vi "Lockin-4461 -Patrick -State -sw_timed_single_pt.vi"() -> ()   [LabVIEW 2013]
uses:
  <vilib>/Analysis/4window.llb/windowTd.ctl
  <vilib>/measure/maspectr.llb/Power Spectrum and PSD Export Mode.ctl
  <vilib>/Utility/error.llb/DialogType.ctl
  <vilib>/Analysis/baseanly.llb/Mean (DBL).vi
  <vilib>/Analysis/2dsp.llb/Decimate (single shot).vi
  <vilib>/Analysis/2dsp.llb/Decimate (single shot, DBL).vi
  <userlib>/_OpenG.lib/array/array.llb/Empty 1D Array (Variant)__ogtk.vi
  <userlib>/_OpenG.lib/array/array.llb/Empty 1D Array (DBL)__ogtk.vi
  <vilib>/measure/maspectr.llb/FFT Power Spectrum and PSD for N Chan.vi
  <vilib>/Waveform/WDTOps.llb/WDT Waveform to XY Pairs DBL.vi
  <vilib>/measure/NI_MAPro.lvlib
  <vilib>/Analysis/NI_AALBase.lvlib
  <vilib>/platform/TimedLoop/XDataNode/XDataNode.xnode
  <vilib>/Platform/TimedLoop/XDataNode/nitl_modes.ctl
  <vilib>/Platform/TimedLoop/XDataNode/XDNodeRunTimeDep.lvlib
  <vilib>/Platform/TimedLoop/XDataNode/wakeup.ctl
  <vilib>/Platform/TimedLoop/XDataNode/timing_clust.ctl
  <vilib>/Analysis/NI_AALPro.lvlib
panel:
  in  "save interval (s)":dbl=300.0
  out "save time":timestamp
  out "Error":bool
  out "Results\n(X, Y, R, Theta, mean)":dbl[][](array[numeric])=[[0.808038444568405, -0.03366600088138751, 0.8087394682565412, -2.3857835167729093, -0.00016707925782300797], [9.627554098594765e-06, 5.490802829917109e-06, 1.1083262770429771e-05, 29.69704943130355, -2.2076368724747004e-05], [-0.00010109394038729712, -3.9229110623141134e-05, 0.00010843849825275628, -158.79145052912693, -4.4533407950990875e-05], [0.00012303597772851785, 8.954846359566259e-06, 0.00012336142463888693, 4.162780801361146, -2.013001476212871e-05], [-0.00010354663772943155, 3.541276214228395e-05, 0.00010943477467247838, 161.11940514883716, -0.0003907411187114377], [-2.8426533993272308e-05, 9.227244974626337e-05, 9.655191772848101e-05, 107.1225864279026, 0.00020962577788662882], [-5.4970263568529676e-05, 3.5314916918015216e-05, 6.533661480150268e-05, 147.28182071959253, -3.9837928959940376e-05], [0.00011632495217069192, 2.1805466214220965e-05, 0.00011835105768151502, 10.617056167129062, 7.22324246932892e-05], [0.808038444568405, -0.03366600088138751, 0.8087394682565412, -2.3857835167729093, 0.0], [9.627554098594765e-06, 5.490802829917109e-06, 1.1083262770429771e-05, 29.69704943130355, 0.0], [-0.00010109394038729712, -3.9229110623141134e-05, 0.00010843849825275628, -158.79145052912693, 0.0], [0.00012303597772851785, 8.954846359566259e-06, 0.00012336142463888693, 4.162780801361146, 0.0], [-0.00010354663772943155, 3.541276214228395e-05, 0.00010943477467247838, 161.11940514883716, 0.0], [-2.8426533993272308e-05, 9.227244974626337e-05, 9.655191772848101e-05, 107.1225864279026, 0.0], [-5.4970263568529676e-05, 3.5314916918015216e-05, 6.533661480150268e-05, 147.28182071959253, 0.0], [0.00011632495217069192, 2.1805466214220965e-05, 0.00011835105768151502, 10.617056167129062, 0.0]] format="%#_3p"
  out "current time":timestamp=timestamp(3547736420.9269166 s since 1904-01-01)
  in  "Channel":dbl min=0.0 max=7.0 step=1.0
  in  "Display":enum16{"X and Y", "R and Theta"}(ring)
  out "Y or Theta":dbl=-0.03366600088138751 caption="Y or Theta: Current (A) or Voltage (V)" format="%.3p"
  out "X or R":dbl=0.808038444568405 caption="X or R: Current (A) or Voltage (V)" format="%#.3p"
  in  "Save Data":bool
  in  "RESET":bool
  in  "EXIT":bool
  in  "path":path=path "C:/Data/lockin"
  in  "Notes":string
  in  "mean":dbl[](array[numeric])=[-7.421439795208782e-05, -0.00022642109497774898, -0.00010801336111838228, -0.0001940739070778859, -0.00016525478307431987, 0.00040119220463992125, -0.0005006815886623466, 0.00022102245437355468]
  in  "Tab Control 2":T1(tab)
  out "Signals Graph 2":waveform(dbl)[](graph)=[{"t0"=timestamp(3547736422.7899165 s since 1904-01-01), "dt"=4.8828125e-06, "Y"=array[2048 elements]}, {"t0"=timestamp(3547736422.7899165 s since 1904-01-01), "dt"=4.8828125e-06, "Y"=array[2048 elements]}, {"t0"=timestamp(3547736422.7899165 s since 1904-01-01), "dt"=4.8828125e-06, "Y"=array[2048 elements]}, {"t0"=timestamp(3547736422.7899165 s since 1904-01-01), "dt"=4.8828125e-06, "Y"=array[2048 elements]}, {"t0"=timestamp(3547736422.7899165 s since 1904-01-01), "dt"=4.8828125e-06, "Y"=array[2048 elements]}, {"t0"=timestamp(3547736422.7899165 s since 1904-01-01), "dt"=4.8828125e-06, "Y"=array[2048 elements]}, {"t0"=timestamp(3547736422.7899165 s since 1904-01-01), "dt"=4.8828125e-06, "Y"=array[2048 elements]}, {"t0"=timestamp(3547736422.7899165 s since 1904-01-01), "dt"=4.8828125e-06, "Y"=array[2048 elements]}]
  out "Signals Graph":waveform(dbl)[](graph)=[{"t0"=timestamp(3547736419.2449164 s since 1904-01-01), "dt"=4.8828125e-05, "Y"=array[20480 elements]}, {"t0"=timestamp(3547736419.2449164 s since 1904-01-01), "dt"=4.8828125e-05, "Y"=array[20480 elements]}, {"t0"=timestamp(3547736419.2449164 s since 1904-01-01), "dt"=4.8828125e-05, "Y"=array[20480 elements]}, {"t0"=timestamp(3547736419.2449164 s since 1904-01-01), "dt"=4.8828125e-05, "Y"=array[20480 elements]}, {"t0"=timestamp(3547736419.2449164 s since 1904-01-01), "dt"=4.8828125e-05, "Y"=array[20480 elements]}, {"t0"=timestamp(3547736419.2449164 s since 1904-01-01), "dt"=4.8828125e-05, "Y"=array[20480 elements]}, {"t0"=timestamp(3547736419.2449164 s since 1904-01-01), "dt"=4.8828125e-05, "Y"=array[20480 elements]}, {"t0"=timestamp(3547736419.2449164 s since 1904-01-01), "dt"=4.8828125e-05, "Y"=array[20480 elements]}]
  out "Reference Graph":waveform(dbl)[](graph)=[{"t0"=timestamp(3547736419.2449164 s since 1904-01-01), "dt"=4.8828125e-05, "Y"=array[20480 elements]}, {"t0"=timestamp(3547736419.2449164 s since 1904-01-01), "dt"=4.8828125e-05, "Y"=array[20480 elements]}, {"t0"=timestamp(3547736419.2449164 s since 1904-01-01), "dt"=4.8828125e-05, "Y"=array[20480 elements]}, {"t0"=timestamp(3547736419.2449164 s since 1904-01-01), "dt"=4.8828125e-05, "Y"=array[20480 elements]}, {"t0"=timestamp(3547736419.2449164 s since 1904-01-01), "dt"=4.8828125e-05, "Y"=array[20480 elements]}, {"t0"=timestamp(3547736419.2449164 s since 1904-01-01), "dt"=4.8828125e-05, "Y"=array[20480 elements]}, {"t0"=timestamp(3547736419.2449164 s since 1904-01-01), "dt"=4.8828125e-05, "Y"=array[20480 elements]}, {"t0"=timestamp(3547736419.2449164 s since 1904-01-01), "dt"=4.8828125e-05, "Y"=array[20480 elements]}]
  in  "decimate graph":i32=1
  in  "Display n?":bool
  out "Display X (or R)":waveform(dbl)[](graph)=[{"t0"=timestamp(3547736419.2449164 s since 1904-01-01), "dt"=1.0, "Y"=[0.808038444568405]}, {"t0"=timestamp(3547736419.2449164 s since 1904-01-01), "dt"=1.0, "Y"=[9.627554098594765e-06]}, {"t0"=timestamp(3547736419.2449164 s since 1904-01-01), "dt"=1.0, "Y"=[-0.00010109394038729712]}, {"t0"=timestamp(3547736419.2449164 s since 1904-01-01), "dt"=1.0, "Y"=[0.00012303597772851785]}, {"t0"=timestamp(3547736419.2449164 s since 1904-01-01), "dt"=1.0, "Y"=[-0.00010354663772943155]}, {"t0"=timestamp(3547736419.2449164 s since 1904-01-01), "dt"=1.0, "Y"=[-2.8426533993272308e-05]}, {"t0"=timestamp(3547736419.2449164 s since 1904-01-01), "dt"=1.0, "Y"=[-5.4970263568529676e-05]}, {"t0"=timestamp(3547736419.2449164 s since 1904-01-01), "dt"=1.0, "Y"=[0.00011632495217069192]}, {"t0"=timestamp(3547736419.2449164 s since 1904-01-01), "dt"=1.0, "Y"=[0.808038444568405]}, {"t0"=timestamp(3547736419.2449164 s since 1904-01-01), "dt"=1.0, "Y"=[9.627554098594765e-06]}, {"t0"=timestamp(3547736419.2449164 s since 1904-01-01), "dt"=1.0, "Y"=[-0.00010109394038729712]}, {"t0"=timestamp(3547736419.2449164 s since 1904-01-01), "dt"=1.0, "Y"=[0.00012303597772851785]}, {"t0"=timestamp(3547736419.2449164 s since 1904-01-01), "dt"=1.0, "Y"=[-0.00010354663772943155]}, {"t0"=timestamp(3547736419.2449164 s since 1904-01-01), "dt"=1.0, "Y"=[-2.8426533993272308e-05]}, {"t0"=timestamp(3547736419.2449164 s since 1904-01-01), "dt"=1.0, "Y"=[-5.4970263568529676e-05]}, {"t0"=timestamp(3547736419.2449164 s since 1904-01-01), "dt"=1.0, "Y"=[0.00011632495217069192]}]
  out "Display Y (or Theta)":waveform(dbl)[](graph)=[{"t0"=timestamp(3547736419.2449164 s since 1904-01-01), "dt"=1.0, "Y"=[-0.03366600088138751]}, {"t0"=timestamp(3547736419.2449164 s since 1904-01-01), "dt"=1.0, "Y"=[5.490802829917109e-06]}, {"t0"=timestamp(3547736419.2449164 s since 1904-01-01), "dt"=1.0, "Y"=[-3.9229110623141134e-05]}, {"t0"=timestamp(3547736419.2449164 s since 1904-01-01), "dt"=1.0, "Y"=[8.954846359566259e-06]}, {"t0"=timestamp(3547736419.2449164 s since 1904-01-01), "dt"=1.0, "Y"=[3.541276214228395e-05]}, {"t0"=timestamp(3547736419.2449164 s since 1904-01-01), "dt"=1.0, "Y"=[9.227244974626337e-05]}, {"t0"=timestamp(3547736419.2449164 s since 1904-01-01), "dt"=1.0, "Y"=[3.5314916918015216e-05]}, {"t0"=timestamp(3547736419.2449164 s since 1904-01-01), "dt"=1.0, "Y"=[2.1805466214220965e-05]}, {"t0"=timestamp(3547736419.2449164 s since 1904-01-01), "dt"=1.0, "Y"=[-0.03366600088138751]}, {"t0"=timestamp(3547736419.2449164 s since 1904-01-01), "dt"=1.0, "Y"=[5.490802829917109e-06]}, {"t0"=timestamp(3547736419.2449164 s since 1904-01-01), "dt"=1.0, "Y"=[-3.9229110623141134e-05]}, {"t0"=timestamp(3547736419.2449164 s since 1904-01-01), "dt"=1.0, "Y"=[8.954846359566259e-06]}, {"t0"=timestamp(3547736419.2449164 s since 1904-01-01), "dt"=1.0, "Y"=[3.541276214228395e-05]}, {"t0"=timestamp(3547736419.2449164 s since 1904-01-01), "dt"=1.0, "Y"=[9.227244974626337e-05]}, {"t0"=timestamp(3547736419.2449164 s since 1904-01-01), "dt"=1.0, "Y"=[3.5314916918015216e-05]}, {"t0"=timestamp(3547736419.2449164 s since 1904-01-01), "dt"=1.0, "Y"=[2.1805466214220965e-05]}]
  out "names":string[](array[string])
  out "XY Graph":cluster{dbl[], dbl[]}[](graph)=[{[0.0, 0.808038444568405], [0.0, -0.03366600088138751]}, {[0.0, 9.627554098594765e-06], [0.0, 5.490802829917109e-06]}, {[0.0, -0.00010109394038729712], [0.0, -3.9229110623141134e-05]}, {[0.0, 0.00012303597772851785], [0.0, 8.954846359566259e-06]}, {[0.0, -0.00010354663772943155], [0.0, 3.541276214228395e-05]}, {[0.0, -2.8426533993272308e-05], [0.0, 9.227244974626337e-05]}, {[0.0, -5.4970263568529676e-05], [0.0, 3.5314916918015216e-05]}, {[0.0, 0.00011632495217069192], [0.0, 2.1805466214220965e-05]}, {[0.0, 0.808038444568405], [0.0, -0.03366600088138751]}, {[0.0, 9.627554098594765e-06], [0.0, 5.490802829917109e-06]}, {[0.0, -0.00010109394038729712], [0.0, -3.9229110623141134e-05]}, {[0.0, 0.00012303597772851785], [0.0, 8.954846359566259e-06]}, {[0.0, -0.00010354663772943155], [0.0, 3.541276214228395e-05]}, {[0.0, -2.8426533993272308e-05], [0.0, 9.227244974626337e-05]}, {[0.0, -5.4970263568529676e-05], [0.0, 3.5314916918015216e-05]}, {[0.0, 0.00011632495217069192], [0.0, 2.1805466214220965e-05]}]
  out "PS Chart":dbl[][](graph)=[[-1411.497616925462, -1404.3790029743438, -1413.0961920610762, -1418.6418791322994, -1413.136726104145, -1413.4151534226191, -1417.9246313001065, -1424.6072395567076]]
  out "PS dB":cluster{"f0":dbl, "df":dbl, "magnitude":dbl[]}[](graph)
  in  "window":T2=1 items=["Rectangle"=0, "Hanning"=1, "Hamming"=2, "Blackman-Harris"=3, "Exact Blackman"=4, "Blackman"=5, "Flat Top"=6, "4 Term B-Harris "=7, "7 Term B-Harris"=8, "Low Sidelobe"=9, "Blackman Nuttall"=11, "Triangle"=30, "Bartlett-Hanning"=31, "Bohman"=32, "Parzen"=33, "Welch"=34, "Kaiser"=60, "Dolph-Chebyshev"=61, "Gaussian"=62]
  in  "averaging parameters":T3={"averaging mode"=enum."RMS averaging", "weighting mode"=enum."Exponential", "number of averages"=10} {"number of averages" min=1}
  in  "restart averaging (F)":bool
  in  "export mode":T4 items=["Power Spectrum", "Power Spectral Density"]
  in  "window parameter":dbl=nan
  out "averages\ncompleted":dbl=8319.0
  out "averaging done":bool=TRUE
  in  "Tab Control":T5(tab)=enum."AO/Lockin Setup"
  in  "decimating factor":i32=10
  in  "AI Buffer Size (S)":i32=100
  out "dt":dbl=4.8828125e-05 format="%#_6p"
  in  "IV curves?\n(not used)":bool
  in  "AO Configuration":T6(array[cluster])=[{"Output physical channels"="PXI1Slot2/ao0:1", "AO. Max"=0.1, "AO.Min"=-0.1}, {"Output physical channels"="PXI1Slot3/ao0:1", "AO. Max"=0.1, "AO.Min"=-0.1}, {"Output physical channels"="PXI1Slot4/ao0:1", "AO. Max"=0.1, "AO.Min"=-0.1}, {"Output physical channels"="PXI1Slot5/ao0:1", "AO. Max"=0.1, "AO.Min"=-0.1}]
  in  "AI Configuration":T7(array[cluster])=[{"AI.Coupling"=10050, "AI.Max"=0.1, "AI.Min"=-0.1, "Input physical channels"="PXI1Slot2/ai0:1"}, {"AI.Coupling"=10050, "AI.Max"=0.1, "AI.Min"=-0.1, "Input physical channels"="PXI1Slot3/ai0:1"}, {"AI.Coupling"=10050, "AI.Max"=0.1, "AI.Min"=-0.1, "Input physical channels"="PXI1Slot4/ai0:1"}, {"AI.Coupling"=10050, "AI.Max"=0.1, "AI.Min"=-0.1, "Input physical channels"="PXI1Slot5/ai0:1"}] {"AI.Coupling" items=["AC"=10045, "DC"=10050, "GND"=10066]}
  out "error":errorcluster
  in  "measure offset":bool
  in  "reset signal":bool
  in  "all  f same?":bool
  in  "reset REF phi to zero":bool
  in  "zero offset":bool
  in  "LP cutoff (Hz)":dbl=10.0
  in  "LP prefilter":bool
  in  "60 Hz prefilter":bool
  in  "Wait on Trigger":bool
  in  "Remote Mode":bool
  in  "Channels: AO":T8={"AO amp (V)"=[1.0, 0.0, 0.0, 0.0, 0.0, 0.0, 0.0, 0.0], "AO DC (V)"=[0.0, 0.0, 0.0, 0.0, 0.0, 0.0, 0.0, 0.0], "AO f (Hz)"=[1.0, 1.0, 1.0, 1.0, 1.0, 1.0, 1.0, 1.0], "AO phi (deg)"=[0.0, 0.0, 0.0, 0.0, 0.0, 0.0, 0.0, 0.0], "function"=[enum."Triangle Wave", enum."Sine Wave", enum."Sine Wave", enum."Sine Wave", enum."Sine Wave", enum."Sine Wave", enum."Sine Wave", enum."Sine Wave"]} {"AO f (Hz)" min=0.001 max=1000.0; "AO DC (V)" format="%#_6p"; "AO amp (V)" format="%#_6p"}
  in  "Channels: Lockin":T9={"REF f (Hz)"=[1.0, 1.0], "REF phi (deg)"=[0.0, 0.0]} {"REF phi (deg)" format="%#_3g"}
  in  "simulate?":bool=TRUE
  in  "order":i32=2
  in  "TC (s)":dbl=1.0
  out "filter fC (Hz)":dbl=0.3183098861837907
  in  "autophase?\n(experimental)":bool
  in  "P":dbl=0.5 format="%.2f"
  in  "I":dbl=0.6 format="%.2f"
  in  "D":dbl=0.019999999999999997 format="%.2f"
  out "time since trigger":dbl
  in  "auto block size":bool
  in  "x":dbl=1000.0 format="%#_13g"
  in  "sampling info":cluster{"Fs":i32, "#s":i32}={"Fs"=204800, "#s"=2048}
  in  "Numeric":i32=100
  in  "offsets":dbl[](array[numeric])=[0.0, 0.0, 0.0, 0.0, 0.0, 0.0, 0.0, 0.0] format="%#.2p"
  in  "Gain":dbl[](array[numeric])=[1.0, 1.0, 1.0, 1.0, 1.0, 1.0, 1.0, 1.0]
  out "phase log":dbl[](array[numeric])=[1007.0, 1007.0, 1007.0, 1007.0, 1007.0, 1007.0, 1007.0, 1007.0] format="%.1f"
  # "´"
  # "Multichannel Lockin v2016/06/02 ............................................."
  # "this is disabled!"
  # "plot 0    = AI0 f0\nplot 1    = Ai1 f0\n...\nplot N-1  = AIN f0\n\nplot N    = AI0 f1\nplot N+1  = AI1 f1\n..."
  # "sampling"
  # "prefilters"
  # "Make fs x*f0"
  # "lockin filter"
  # "autophase"
  # "0"
  # "1"
  # "2"
  # "3"
  # "4"
  # "5"
  # "6"
  # "7"
  # "Random Thoughts\n1. change the path in the yellow box below where you want to save the signal traces for diagnostics\n(G:\\ on CustardPie, H:\\ on WindySea)\n2. Change the AI and AO limits on the DAQ Settings tab\n\nPlease email p.irvin@levylab.org with questions or suggestions. Thanks."
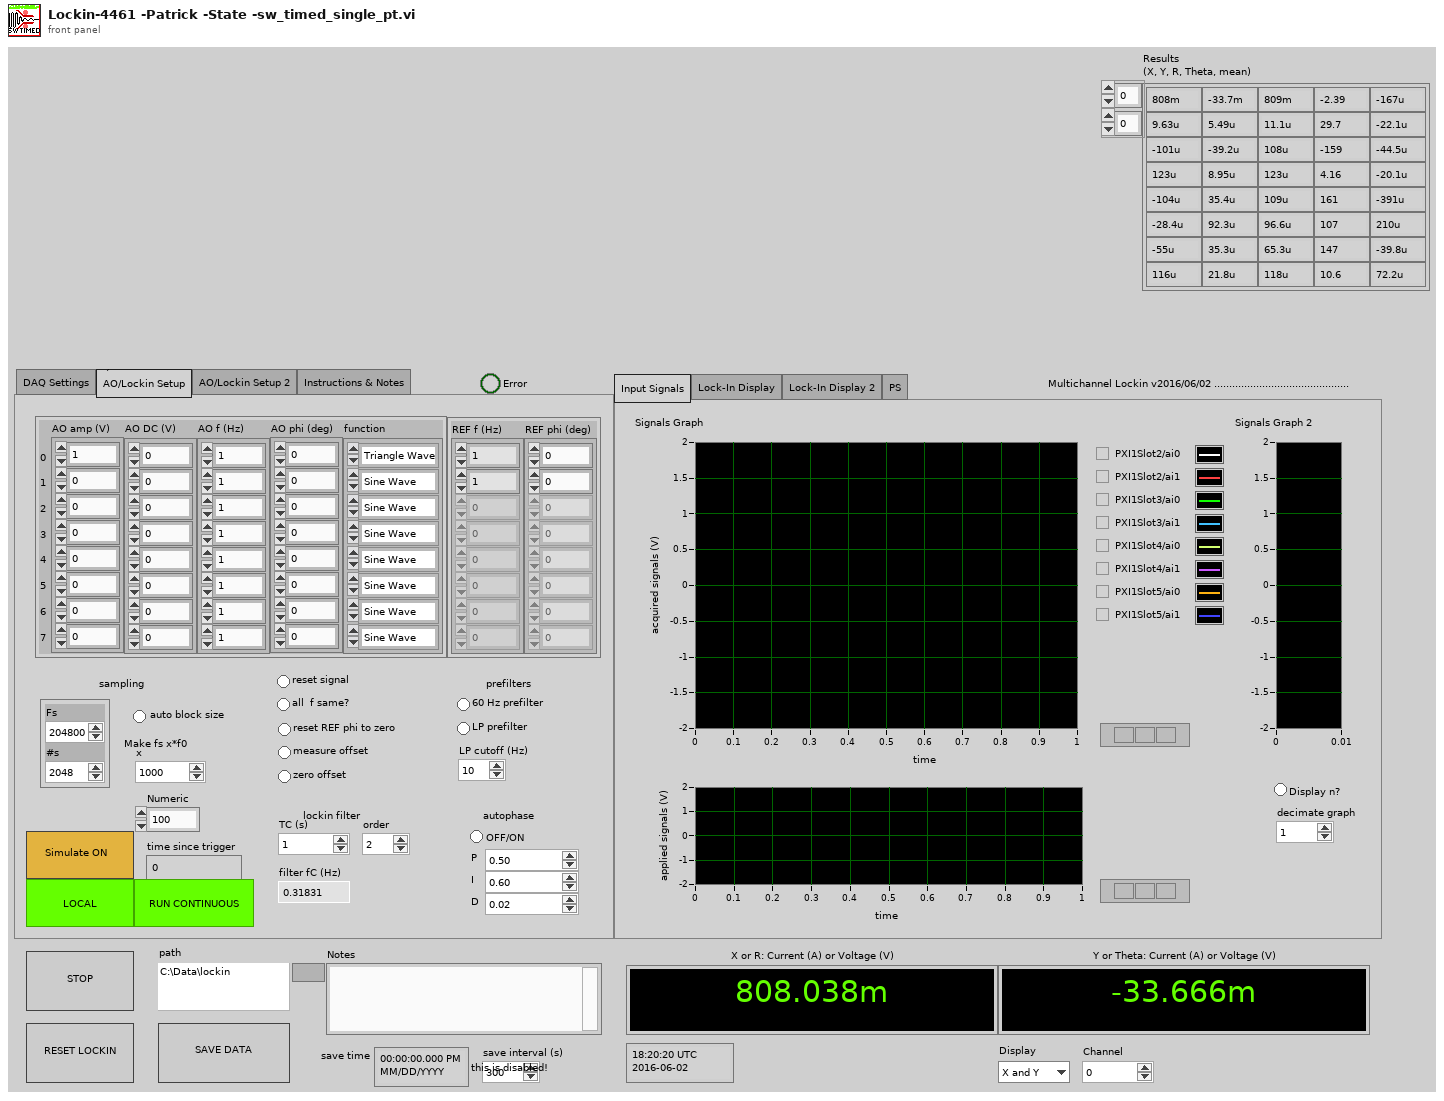
[diagram p1: front panel]
types:
  T1 = enum32{"Input Signals", "Lock-In Display", "Lock-In Display 2", "PS"}
  T2 = typedef "NI_AALPro.lvlib/windowTd.ctl" = u32
  T3 = cluster{"averaging mode":enum16{"No averaging", "Vector averaging", "RMS averaging", "Peak hold"}, "weighting mode":enum16{"Linear", "Exponential"}, "number of averages":u32}
  T4 = typedef "NI_MAPro.lvlib/Power Spectrum and PSD Export Mode.ctl" = u16
  T5 = enum32{"DAQ Settings", "AO/Lockin Setup", "AO/Lockin Setup 2", "Instructions & Notes"}
  T6 = cluster{"Output physical channels":tag, "AO. Max":dbl, "AO.Min":dbl}[]
  T7 = cluster{"AI.Coupling":i32, "AI.Max":dbl, "AI.Min":dbl, "Input physical channels":tag}[]
  T8 = cluster{"AO amp (V)":dbl[], "AO DC (V)":dbl[], "AO f (Hz)":dbl[], "AO phi (deg)":dbl[], "function":enum16{"Sine Wave", "Triangle Wave", "Square Wave", "Sawtooth Wave"}[]}
  T9 = cluster{"REF f (Hz)":dbl[], "REF phi (deg)":dbl[]}
  T10 = typedef "XDNodeRunTimeDep.lvlib/timing_clust.ctl" = cluster{"Expected End [f-1]":u64, "Actual End [f-1]":u64, "Finished Late? [f-1]":bool, "Expected End [i-1]":u64, "Actual End [i-1]":u64, "Finished Late? [i-1]":bool, "Expected Start [i]":u64, "Actual Start [i]":u64, "Expected Start [f]":u64, "Actual Start [f]":u64, "Source Name":string, "Structure Name":string, "Period":i64, "Deadline":i64, "Offset":i64, "Start":i64, "Priority":i32, "Timeout":i32, "Mode":T11, "Wakeup Reason":T12, "Error":errorcluster, "Source Type":string, "Secondary Source Type":string, "Global End Time":u64, "Global Start Time":u64, "Frame Duration":u64, "Iteration Duration":u64, "Assigned CPU":i32, "I/O Scan Engine Mode":u32}
  T11 = typedef "XDNodeRunTimeDep.lvlib/nitl_modes.ctl" = enum32{"No Change", "Process missed periods, maintain original phase", "Discard missed periods, maintain original phase", "Process missed periods, ignore original phase", "Discard missed periods, ignore original phase"}
  T12 = typedef "XDNodeRunTimeDep.lvlib/wakeup.ctl" = enum32{"Normal", "Aborted", "Asynchronous wakeup", "Timing source error", "Timed loop error", "Timeout"}
  T13 = enum32{"invalid app kind", "Development System", "Run Time System", "Student Edition", "Embedded LabVIEW", "Evaluation", "Custom"}
  T14 = enum32{"Invalid", "Standard", "Closed", "Hidden", "Minimized", "Maximized"}
  T15 = enum32{"Input Signals", "Lock-In Display", "Lock-In Display 2", "PS", "FFT"}
  T16 = cluster{"Core":cluster{"Current VI Reference":refnum<vi>, "Close Panel on Exit?":bool}, "Error":bool, "Your string data":string, "AI task":refnum<k21>[], "AO task":refnum<k21>[], "Input Signals":waveform(dbl)[], "Ouput Signals":waveform(dbl)[], "REF":waveform(dbl)[], "sampling info":cluster{"Fs":dbl, "#s":dbl}}
  T17 = typedef "DialogType.ctl" = u16
  T18 = cluster{"Current VI Reference":refnum<vi>, "Close Panel on Exit?":bool}
  T19 = cluster{"AO amp (V)":bool[], "AO DC (V)":bool[], "AO f (Hz)":bool[], "AO phi (deg)":bool[], "function":bool[]}
  T20 = cluster{"REF f (Hz)":bool[], "REF phi (deg)":bool[]}
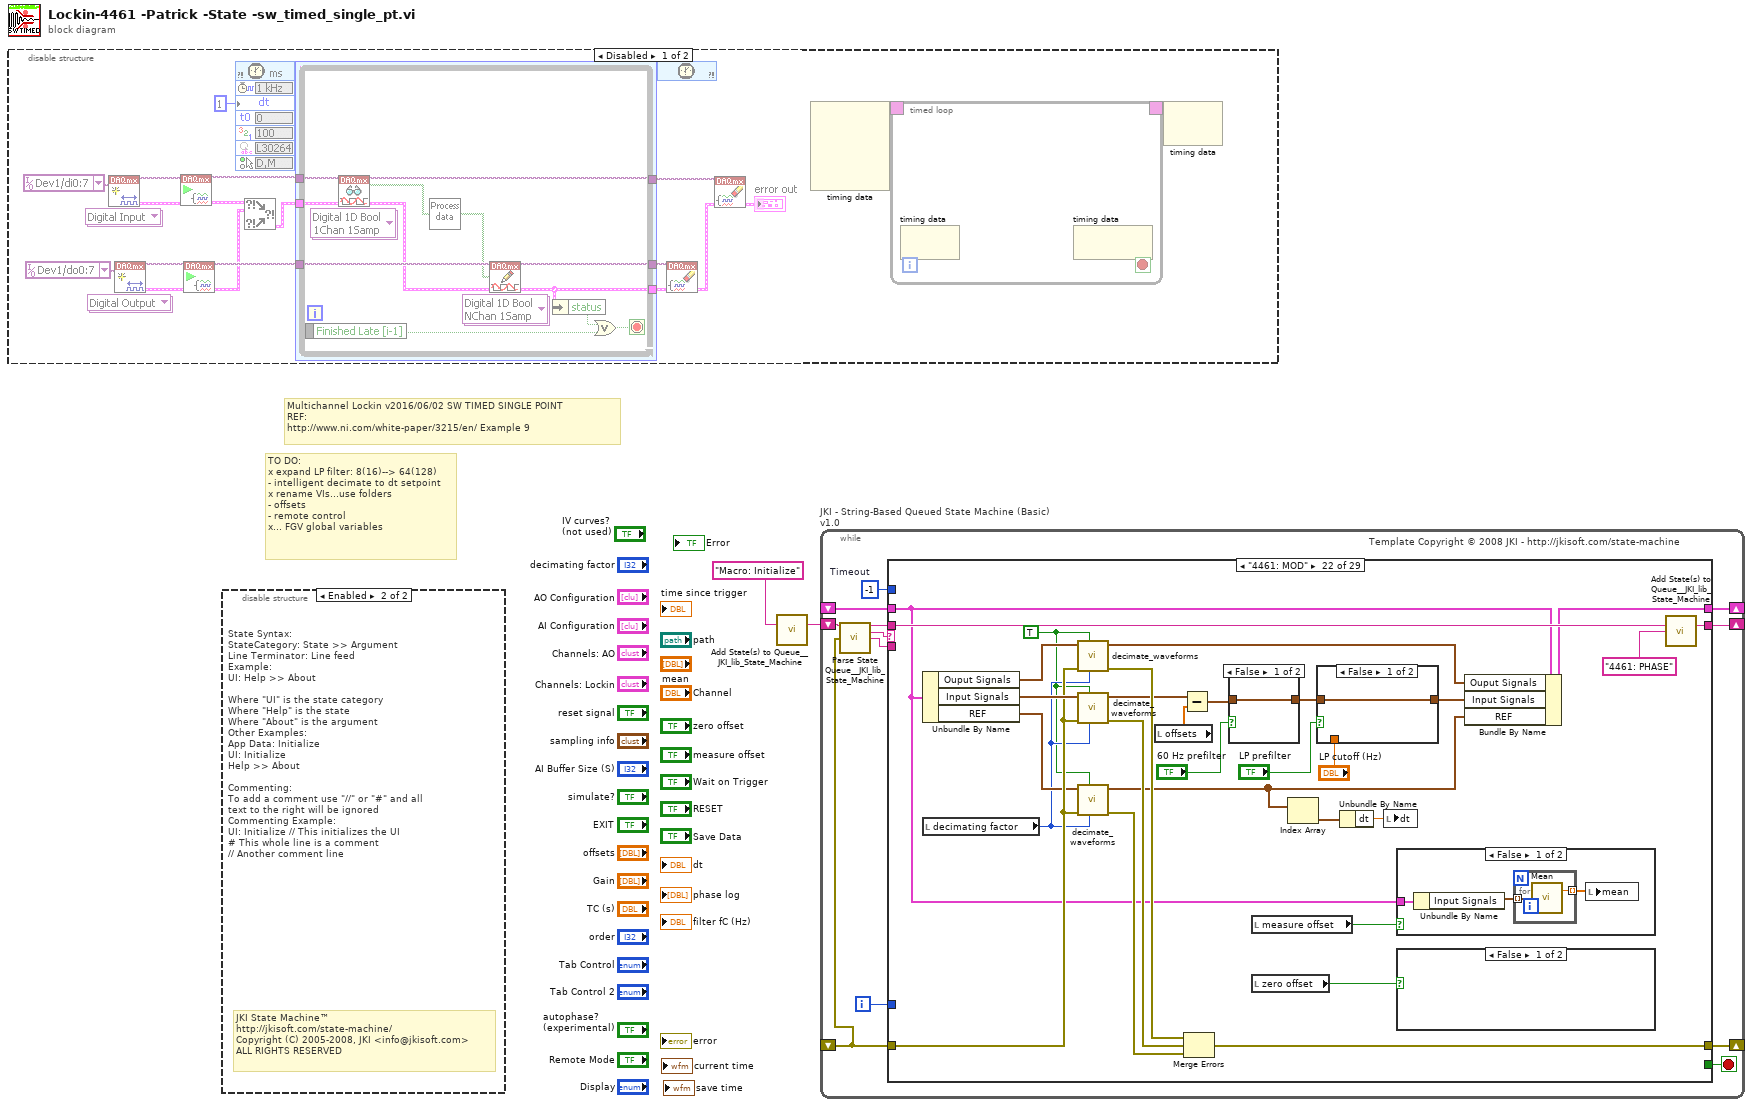
[diagram p0: block diagram]
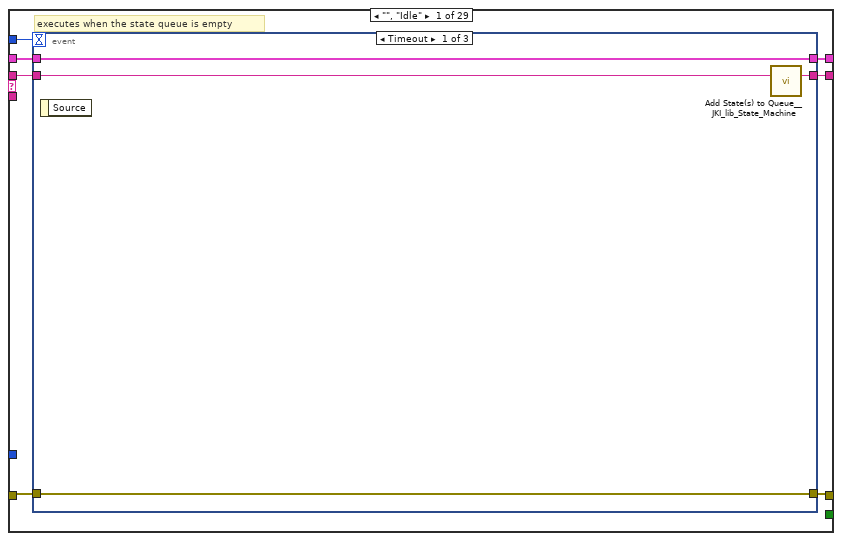
[diagram p4: hidden frame]
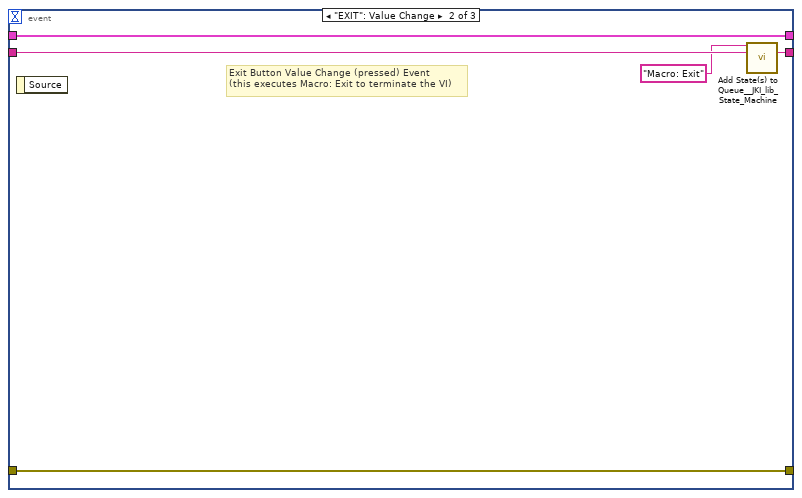
[diagram p5: hidden frame]
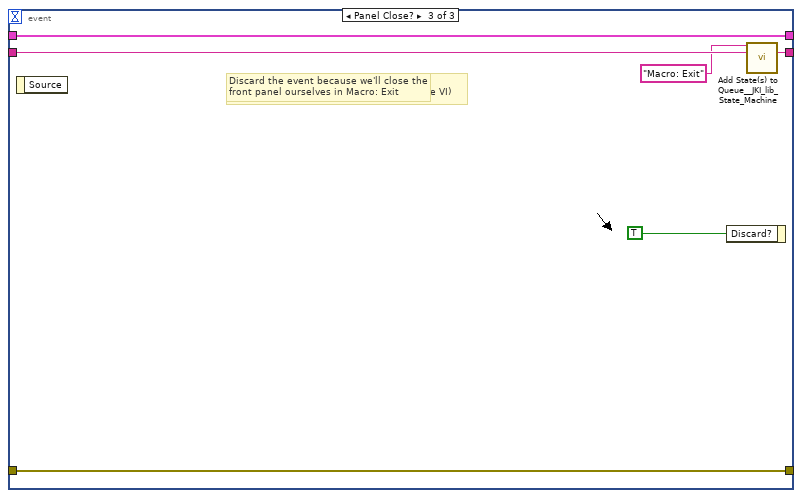
[diagram p6: hidden frame]
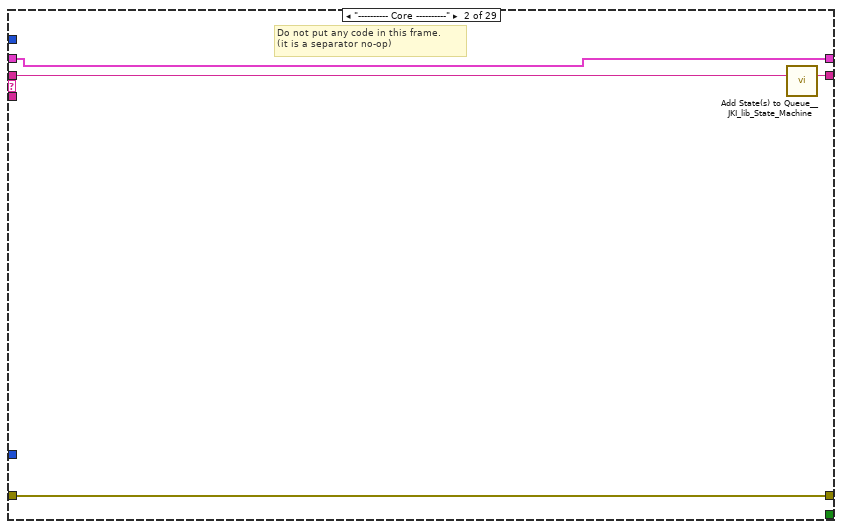
[diagram p7: hidden frame]
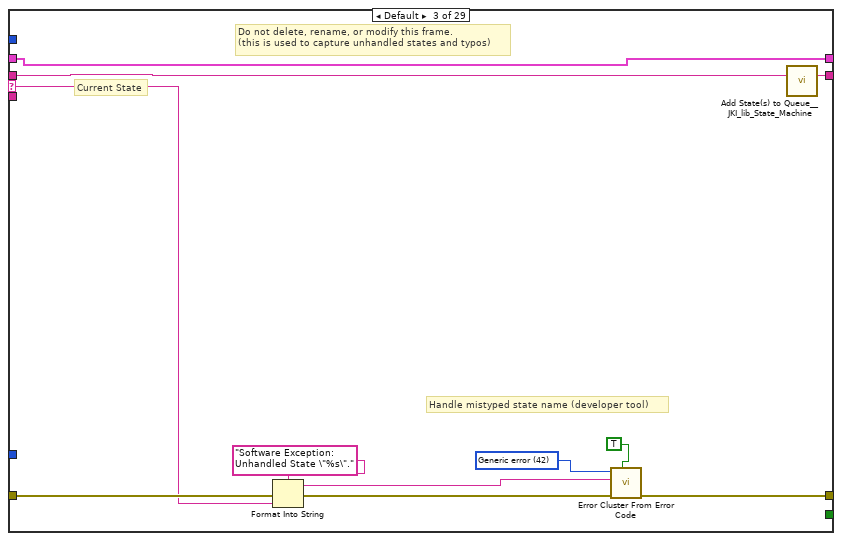
[diagram p8: hidden frame]
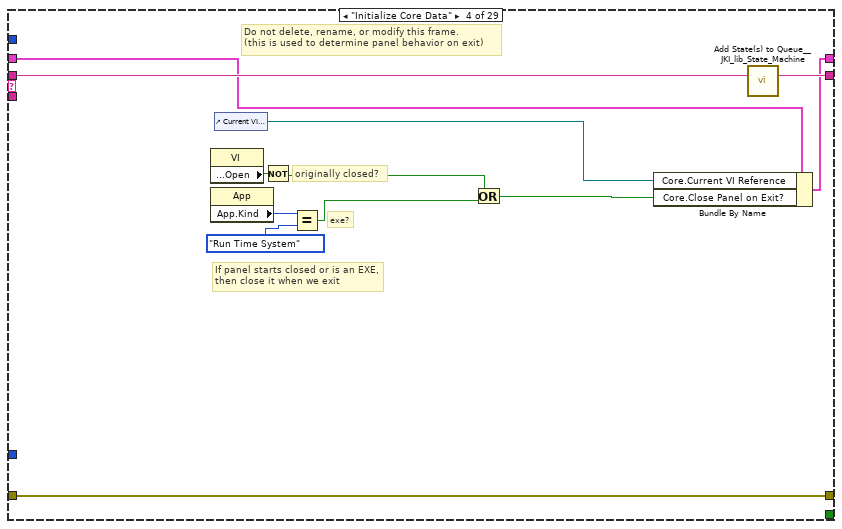
[diagram p9: hidden frame]
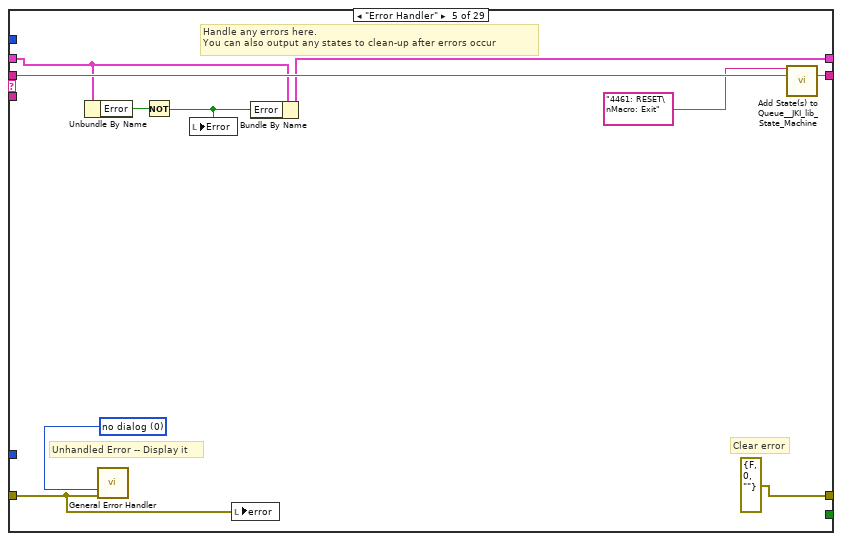
[diagram p10: hidden frame]
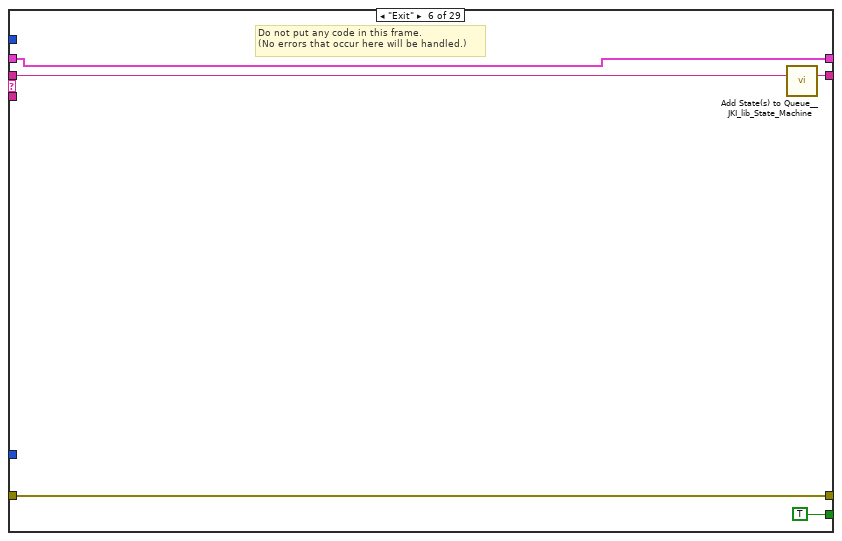
[diagram p11: hidden frame]
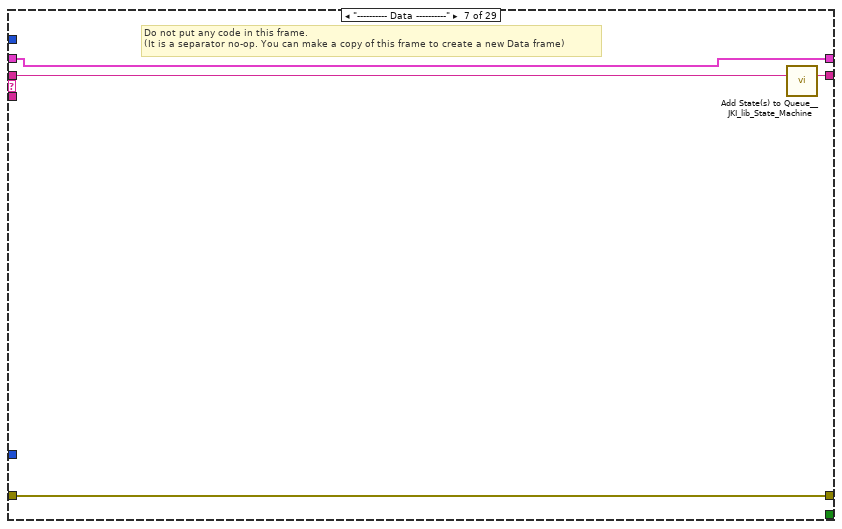
[diagram p12: hidden frame]
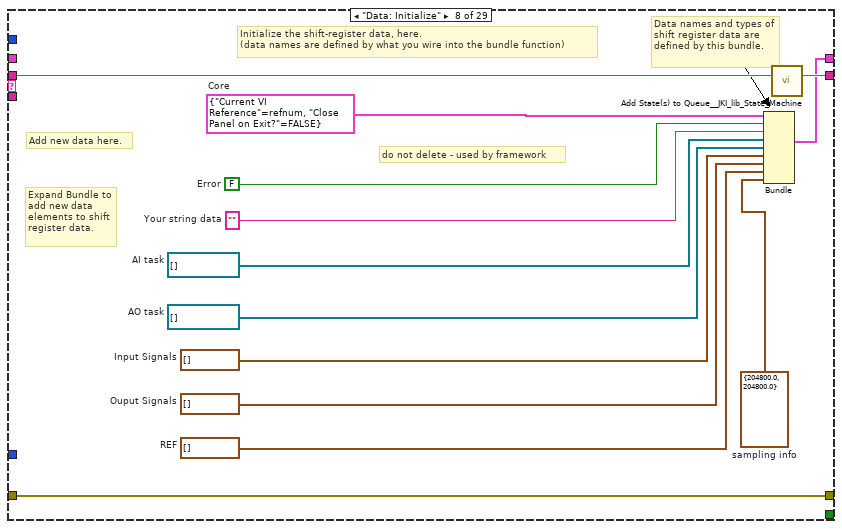
[diagram p13: hidden frame]
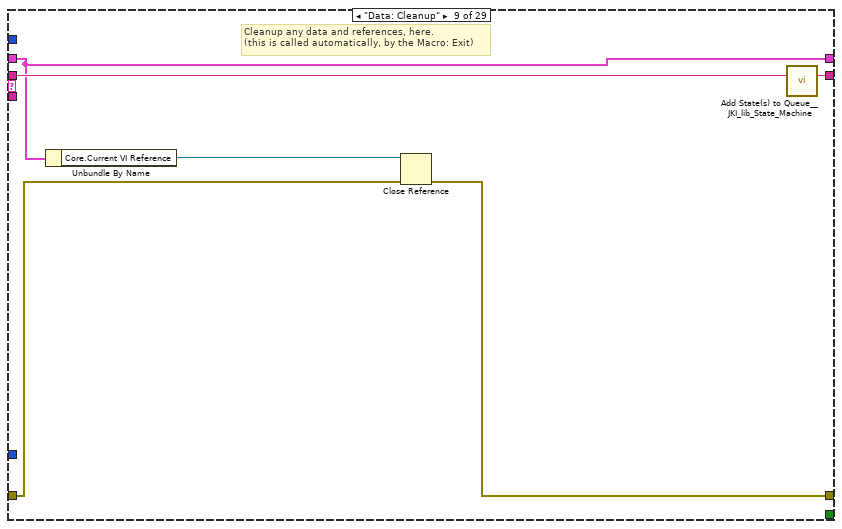
[diagram p14: hidden frame]
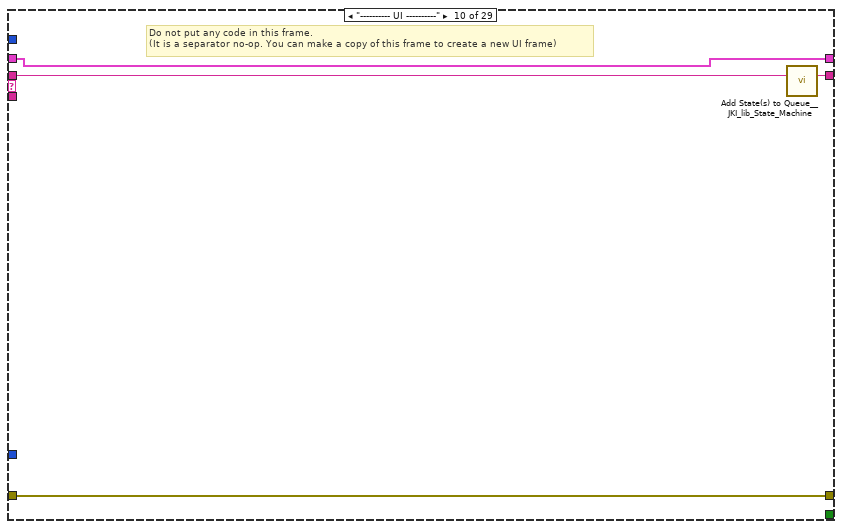
[diagram p15: hidden frame]
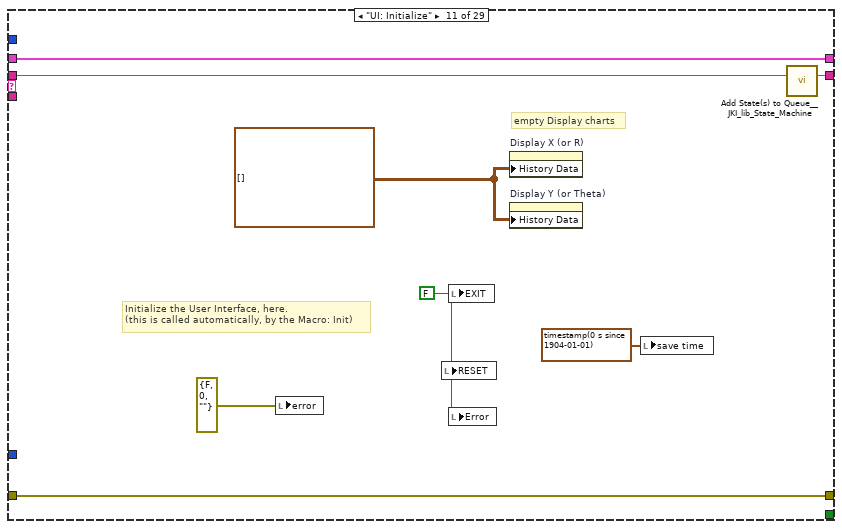
[diagram p16: hidden frame]
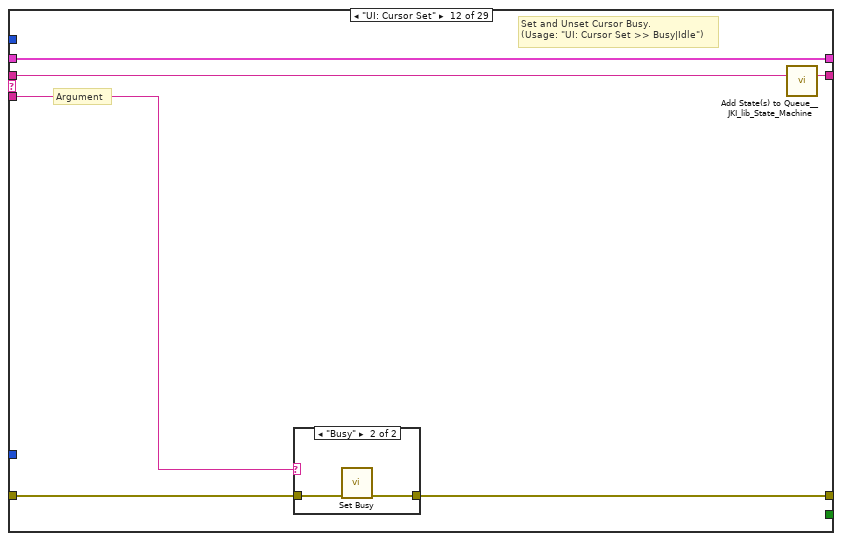
[diagram p17: hidden frame]
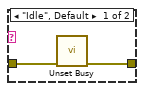
[diagram p18: hidden frame]
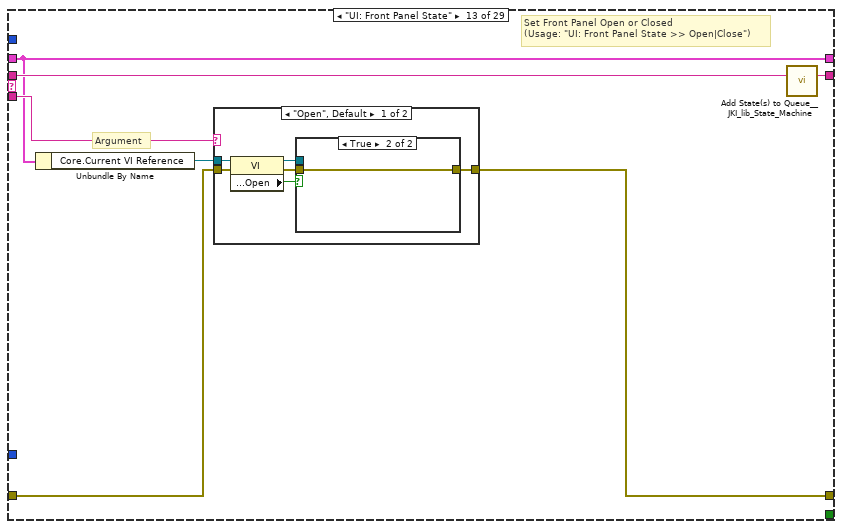
[diagram p19: hidden frame]
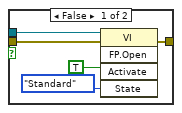
[diagram p20: hidden frame]
diagram:
  # "Multichannel Lockin v2016/06/02 SW TIMED SINGLE POINT\nREF:\nhttp://www.ni.com/white-paper/3215/en/ Example 9"
  # "TO DO:\nx expand LP filter: 8(16)--> 64(128)\n- intelligent decimate to dt setpoint\nx rename VIs...use folders\n- offsets\n- remote control\nx... FGV global variables"
  n1 = disable-structure shown="Disabled" {
    frame Disabled {
      n2 = node-c288() -> (w4:T10)  [unwired: 4 in]
      n3 = timed-loop {
        timing: w4 -> [_]
        timing-out: [_] -> w3
        stop <- _ stop-if-true
        n4 = node-c288() -> ()  [unwired: 1 in, 1 out]
        n5 = node-c288() -> ()  [unwired: 1 in, 1 out]
      }
      n6 = node-c288(w3) -> ()  [unwired: 1 out]
    }
    frame Enabled {
    }
  }
  n7 = disable-structure shown="Enabled" {
    frame Disabled {
    }
    frame Enabled {
      # "JKI State Machine™\nhttp://jkisoft.com/state-machine/\nCopyright (C) 2005-2008, JKI <info@jkisoft.com>\nALL RIGHTS RESERVED"
      # "State Syntax:\nStateCategory: State >> Argument\nLine Terminator: Line feed\nExample:\nUI: Help >> About\n\nWhere \"UI\" is the state category\nWhere \"Help\" is the state\nWhere \"About\" is the argument\nOther Examples:\nApp Data: Initialize\nUI: Initialize\nHelp >> About\n\nCommenting:\nTo add a comment use \"//\" or \"#\" and all text to the right will be ignored\nCommenting Example:\nUI: Initialize // This initializes the UI\n# This whole line is a comment\n// Another comment line"
    }
  }
  n8 = call <vilib>:"Add State(s) to Queue__JKI_lib_State_Machine.vi"("State(s) in (\"\")"="Macro: Initialize") -> ("States Out"=w2:string)  [unwired: 14 in]
  n9 = while "JKI - String-Based Queued State Machine (Basic) v1.0" {
    shift-right: [w14] -> _
    shift-left: _ -> [w13]
    shift-right: [w17] -> _
    shift-left: _ -> [w11]
    shift-right: [w16] -> _
    shift-left: w2 -> [w18]
    i -> [w9]
    stop <- w15 stop-if-true
    w12 = -1  # Timeout
    # "Template Copyright © 2008 JKI - http://jkisoft.com/state-machine"
    n10 = call <vilib>:"Parse State Queue__JKI_lib_State_Machine.vi"("State Queue"=w18, "Error In (no error)"=w11) -> ("Remaining States"=w10:string, "Current State"=w20:string, "Arguments"=w19:string)  [unwired: 11 in]
    n11 = case shown="\"4461: MOD\"" w20 {
      selector: w20 -> [_ _ w47 _ _ _ _ _ _ _ _ _ _ _ _ _ _ _ _ _ _ _ _ _ _ _ _ _ _]
      tunnel: w19 -> [_ _ _ _ _ _ _ _ _ _ _ w121 w132 _ _ _ _ _ _ _ _ _ _ _ _ _ _ _ _]
      tunnel: w13 -> [w25 w43 w49 w60 w72 w82 w85 _ w102 w108 w116 w120 w131 w159 w163 w168 w179 w187 w230 w306 w331 w411 w470 w491 w599 w633 w672 w707 w747]
      tunnel: [w24 w44 w53 w66 errorcluster {"status"=FALSE, "code"=0, "source"=""} ("error out") w81 w86 w98 w103 w109 w114 w122 w130 w160 w165 w176 w180 w197 w232 w299 w341 w425 w459 w488 w601 w627 w662 w701 w745] -> w17
      tunnel: w11 -> [w23 w44 w52 w66 w74 w81 w86 w98 w104 w109 w114 w123 w134 w160 w165 w176 w180 w193 w236 w295 w343 w428 w459 w489 w601 w629 w661 w702 w746]
      tunnel: [w26 w45 w50 w68 w78 w83 w87 w100 w106 w110 w118 w124 w135 w161 w166 w177 w181 w208 w243 w305 w345 w436 w471 w487 w600 w634 w673 w703 w751] -> w16
      tunnel: [_ _ _ _ _ TRUE _ _ _ _ _ _ _ _ _ _ _ _ _ _ _ _ _ _ _ _ _ _ _] -> w15
      tunnel: [w22 w43 w49 w67 w71 w82 w85 w99 w102 w108 w116 w120 w131 w159 w163 w168 w179 w185 w238 w306 w344 w435 w470 w486 w599 w633 w672 w707 w747] -> w14
      tunnel: w12 -> [w21 _ _ _ _ _ _ _ _ _ _ _ _ _ _ _ _ _ _ _ _ _ _ _ _ _ _ _ _]
      tunnel: w10 -> [w27 w46 w51 w69 w79 w84 w88 w101 w107 w111 w119 w125 w136 w162 w167 w178 w182 w209 w244 w304 w346 w437 w472 w490 w602 w635 w674 w705 w751]
      tunnel: w9 -> [_ _ _ _ _ _ _ _ _ _ _ _ _ _ _ _ _ _ _ _ _ _ _ _ _ _ _ _ w750]
      frame "", "Idle" {
        # "executes when the state queue is empty"
        n12 = event shown="[0] Timeout" {
          selector: _ -> [_ _ _]
          dyn-events: _ -> [_ _ _]
          timeout: w21 -> [_ _ _]
          tunnel: w27 -> [w31 w36 w42]
          tunnel: [w30 w35 w41] -> w26
          tunnel: w25 -> [w28 w33 w39]
          tunnel: [w29 w34 w40] -> w24
          tunnel: w23 -> [w29 w34 w40]
          tunnel: [w28 w33 w39] -> w22
          event Timeout {
            n13 = event-data() -> ()  [unwired: 1 in, 1 out]
            n14 = call <vilib>:"Add State(s) to Queue__JKI_lib_State_Machine.vi"("State(s) in (\"\")"=w31) -> ("States Out"=w30:string)  [unwired: 14 in]
          }
          event "EXIT": Value Change {
            # "Exit Button Value Change (pressed) Event\n(this executes Macro: Exit to terminate the VI)"
            n15 = event-data() -> ()  [unwired: 1 in, 1 out]
            n16 = call <vilib>:"Add State(s) to Queue__JKI_lib_State_Machine.vi"("State(s) in Front (\"\")"="Macro: Exit", "State(s) in (\"\")"=w36) -> ("States Out"=w35:string)  [unwired: 13 in]
          }
          event Panel Close? {
            # "Discard the event because we'll close the front panel ourselves in Macro: Exit"
            # "Close Panel button (pressed) Event\n(this executes Macro: Exit to terminate the VI)"
            n17 = event-data() -> ()  [unwired: 1 in, 1 out]
            n18 = event-data("Discard?"=TRUE) -> ()  [unwired: 1 in, 1 out]
            n19 = call <vilib>:"Add State(s) to Queue__JKI_lib_State_Machine.vi"("State(s) in Front (\"\")"="Macro: Exit", "State(s) in (\"\")"=w42) -> ("States Out"=w41:string)  [unwired: 13 in]
          }
        }
      }
      frame "---------- Core ----------" {
        # "Do not put any code in this frame.\n(it is a separator no-op)"
        n20 = call <vilib>:"Add State(s) to Queue__JKI_lib_State_Machine.vi"("State(s) in (\"\")"=w46) -> ("States Out"=w45:string)  [unwired: 14 in]
      }
      frame Default {
        w56 = 42 items=["No error", "Argument error", "Memory is full", "Out of zone", "End of file", "File already open", "Generic file I/O error", "File not found", "File permission error", "Disk is full", "Duplicate path", "Too many files open", "System feature not enabled", "Resource file not found", "Cannot add resource", "Resource not found", "Image not found", "Image memory error", "Pen does not exist", "Config type invalid", "Config token not found", "Config parse error", "Config memory error", "Bad external code format", "Bad external code offset", "External code not present", "Null window", "Destroy window error", "Null menu", "Print aborted", "Bad print record", "Print driver error", "Windows error during printing", "Memory error during printing", "Print dialog error", "Generic print error", "Invalid device refnum", "Device not found", "Device parameter error", "Device unit error", "Cannot open device", "Device call aborted", "Generic error", "Cancelled by user", "Object ID too low", "Object ID too high", "Object not in heap", "Unknown heap", "Unknown object (invalid DefProc)", "Unknown object (DefProc not in table)", "Message out of range", "Invalid (null) method", "Unknown message", "Manager call not supported", "Bad address", "Network operation in progress", "Network operation timed out", "Connection is busy", "Network attribute not supported", "Network error", "Address in use", "System out of memory", "Connection aborted", "Connection refused", "Not connected", "Already connected", "Connection closed", "Initialization error (interapplication manager)", "Bad occurrence", "Wait on unbound occurrence handler", "Occurrence queue overflow", "Datalog type conflict", "Unused", "Unrecognized type (interapplication manager)", "Memory corrupt", "Failed to make temporary DLL", "Old CIN version", "Drag socket not found", "Failed to load drop-object", "Failed to register OLE object", "Failed to release OLE object", "Format specifier type mismatch", "Unknown format specifier", "Too few format specifiers", "Too many format specifiers", "Scan failed", "Newer CIN version", "Error converting to variant", "Runtime menu error", "Password tampered", "Variant attribute not found", "Incompatible variant data type", "Event data is not available", "Event Store is not present", "Occurrence is not found", "Event Queue is not created", "Event info is not available", "Refnum passed is NULL", "Error retrieving Class GUID", "Error retrieving CoClass GUID", "Error retrieving TypeLib GUID.", "Bad built application magic bytes.", "Specific driver is different from the specific driver associated with the Logical Name.", "There is no session opened to the class driver.", "Max Error", "MAX - Error with config objects", "MAX - Error loading configuration", "MAX - Group not supported"]
        # "Current State"
        # "Do not delete, rename, or modify this frame.\n(this is used to capture unhandled states and typos)"
        # "Handle mistyped state name (developer tool)"
        n21 = Format Into String(format string="Software Exception: Unhandled State \"%s\"." ("message"), error in=w52, w47) -> (resulting string=w55:string, error out=w54:errorcluster)  [unwired: 1 in]
        n22 = call <vilib>:"Error Cluster From Error Code.vi"("show call chain? (False)"=TRUE, "error in (no error)"=w54, "error message (\"\")"=w55, "error code (0)"=w56) -> ("error out"=w53:errorcluster)  [unwired: 5 in]
        n23 = call <vilib>:"Add State(s) to Queue__JKI_lib_State_Machine.vi"("State(s) in (\"\")"=w51) -> ("States Out"=w50:string)  [unwired: 14 in]
      }
      frame "Initialize Core Data" {
        # "Do not delete, rename, or modify this frame.\n(this is used to determine panel behavior on exit)"
        # "originally closed?"
        # "exe?"
        # "If panel starts closed or is an EXE, then close it when we exit"
        n24 = property class="VI"() -> ("Front Panel.Open"=w65:bool)  [unwired: 2 in, 2 out]
        n25 = property class="App"() -> ("App.Kind"=w64:T13)  [unwired: 2 in, 2 out]
        n26 = control-ref of="Current VI Reference"() -> (w58:refnum<vi>)
        n27 = Not(x=w65) -> (.not. x?=w62:bool)
        n28 = Equal?(x=w64, y=T13."Run Time System" ("Application:Kind")) -> (x = y?=w61:bool)
        n29 = Or(x=w62, y=w61) -> (x .or. y?=w59:bool)
        n30 = Bundle By Name(cluster=w60, "Core.Current VI Reference"=w58, "Core.Close Panel on Exit?"=w59) -> (w67:T16)
        n31 = call <vilib>:"Add State(s) to Queue__JKI_lib_State_Machine.vi"("State(s) in (\"\")"=w69) -> ("States Out"=w68:string)  [unwired: 14 in]
      }
      frame "Error Handler" {
        w75 = T17 0 items=["no dialog", "OK message", "continue or stop message", "OK message + warnings", "continue/stop + warnings"] ("type of dialog (OK msg:1)")
        # "Unhandled Error -- Display it"
        # "Handle any errors here.\nYou can also output any states to clean-up after errors occur"
        # "Clear error"
        n32 = Unbundle By Name(w72) -> ("Error"=w73:bool)
        n33 = call <vilib>:"General Error Handler.vi"("type of dialog (OK msg:1)"=w75, "error in (no error)"=w74) -> ()  [unwired: 9 in, 5 out]
        n34 = Not(x=w73) -> (.not. x?=w70:bool)
        n35 = local write "Error"(w70) -> ()
        n36 = local write "error"(w74) -> ()
        n37 = Bundle By Name(cluster=w72, "Error"=w70) -> (w71:T16)
        n38 = call <vilib>:"Add State(s) to Queue__JKI_lib_State_Machine.vi"("State(s) in Front (\"\")"="4461: RESET\nMacro: Exit", "State(s) in (\"\")"=w79) -> ("States Out"=w78:string)  [unwired: 13 in]
      }
      frame "Exit" {
        # "Do not put any code in this frame.\n(No errors that occur here will be handled.)"
        n39 = call <vilib>:"Add State(s) to Queue__JKI_lib_State_Machine.vi"("State(s) in (\"\")"=w84) -> ("States Out"=w83:string)  [unwired: 14 in]
      }
      frame "---------- Data ----------" {
        # "Do not put any code in this frame.\n(It is a separator no-op. You can make a copy of this frame to create a new Data frame)"
        n40 = call <vilib>:"Add State(s) to Queue__JKI_lib_State_Machine.vi"("State(s) in (\"\")"=w88) -> ("States Out"=w87:string)  [unwired: 14 in]
      }
      frame "Data: Initialize" {
        w89 = cluster{"Fs":dbl, "#s":dbl} {"Fs"=204800.0, "#s"=204800.0}  # sampling info
        w90 = waveform(dbl)[] []  # Ouput Signals
        w92 = waveform(dbl)[] []  # Input Signals
        w91 = waveform(dbl)[] []  # REF
        w93 = refnum<k21>[] []  # AO task
        w94 = refnum<k21>[] []  # AI task
        w95 = T18 {"Current VI Reference"=refnum, "Close Panel on Exit?"=FALSE}  # Core
        w97 = FALSE  # Error
        w96 = ""  # Your string data
        # "do not delete - used by framework"
        # "Expand Bundle to add new data elements to shift register data."
        # "Add new data here."
        # "Data names and types of shift register data are defined by this bundle."
        # "Initialize the shift-register data, here.\n(data names are defined by what you wire into the bundle function)"
        n41 = Bundle("Core"=w95, "Error"=w97, "Your string data"=w96, "AI task"=w94, "AO task"=w93, "Input Signals"=w92, "Ouput Signals"=w90, "REF"=w91, "sampling info"=w89) -> (w99:T16)  [unwired: 1 in]
        n42 = call <vilib>:"Add State(s) to Queue__JKI_lib_State_Machine.vi"("State(s) in (\"\")"=w101) -> ("States Out"=w100:string)  [unwired: 14 in]
      }
      frame "Data: Cleanup" {
        # "Cleanup any data and references, here.\n(this is called automatically, by the Macro: Exit)"
        n43 = Unbundle By Name(w102) -> ("Core.Current VI Reference"=w105:refnum<vi>)
        n44 = Close Reference(reference=w105, error in (no error)=w104) -> (error out=w103:errorcluster)
        n45 = call <vilib>:"Add State(s) to Queue__JKI_lib_State_Machine.vi"("State(s) in (\"\")"=w107) -> ("States Out"=w106:string)  [unwired: 14 in]
      }
      frame "---------- UI ----------" {
        # "Do not put any code in this frame.\n(It is a separator no-op. You can make a copy of this frame to create a new UI frame)"
        n46 = call <vilib>:"Add State(s) to Queue__JKI_lib_State_Machine.vi"("State(s) in (\"\")"=w111) -> ("States Out"=w110:string)  [unwired: 14 in]
      }
      frame "UI: Initialize" {
        w113 = FALSE ("EXIT")
        w117 = waveform(dbl)[][] [] ("History Data")
        # "empty Display charts"
        # "Initialize the User Interface, here.\n(this is called automatically, by the Macro: Init)"
        n47 = local write "error"(errorcluster {"status"=FALSE, "code"=0, "source"=""} ("error out")) -> ()
        n48 = local write "RESET"(w113) -> ()
        n49 = local write "EXIT"(w113) -> ()
        n50 = local write "Error"(w113) -> ()
        n51 = property on="Display X (or R)" class="WaveformChart (strict)"("History Data"=w117) -> ()  [unwired: 2 in, 2 out]
        n52 = property on="Display Y (or Theta)" class="WaveformChart (strict)"("History Data"=w117) -> ()  [unwired: 2 in, 2 out]
        n53 = local write "save time"(timestamp(0 s since 1904-01-01) ("save time")) -> ()
        n54 = call <vilib>:"Add State(s) to Queue__JKI_lib_State_Machine.vi"("State(s) in (\"\")"=w119) -> ("States Out"=w118:string)  [unwired: 14 in]
      }
      frame "UI: Cursor Set" {
        # "Argument"
        # "Set and Unset Cursor Busy.\n(Usage: \"UI: Cursor Set >> Busy|Idle\")"
        n55 = case shown="\"Busy\"" w121 {
          tunnel: w123 -> [w127 w129]
          tunnel: [w126 w128] -> w122
          frame "Idle", Default {
            n56 = call <vilib>:"Unset Busy.vi"("error in (no error)"=w127) -> ("error out"=w126:errorcluster)  [unwired: 10 in]
          }
          frame "Busy" {
            n57 = call <vilib>:"Set Busy.vi"("error in (no error)"=w129) -> ("error out"=w128:errorcluster)  [unwired: 9 in, 1 out]
          }
        }
        n58 = call <vilib>:"Add State(s) to Queue__JKI_lib_State_Machine.vi"("State(s) in (\"\")"=w125) -> ("States Out"=w124:string)  [unwired: 14 in]
      }
      frame "UI: Front Panel State" {
        # "Argument"
        # "Set Front Panel Open or Closed\n(Usage: \"UI: Front Panel State >> Open|Close\")"
        n59 = Unbundle By Name(w131) -> ("Core.Current VI Reference"=w133:refnum<vi>)
        n60 = case shown="\"Open\", Default" w132 {
          tunnel: w134 -> [w140 w153]
          tunnel: [w142 w154] -> w130
          tunnel: w133 -> [w141 w151]
          frame "Open", Default {
            n61 = property class="VI"(reference=w141, error in=w140) -> (reference out=w138:refnum<vi>, error out=w139:errorcluster, "Front Panel.Open"=w137:bool)
            n62 = case shown="True" w137 {
              tunnel: [w145 w148] -> w142
              tunnel: w139 -> [w144 w148]
              tunnel: w138 -> [w143 _]
              frame False {
                n63 = invoke class="VI" method="FP.Open"(reference=w143, error in=w144, "Activate"=TRUE, "State"=T14."Standard") -> (error out=w145:errorcluster)  [unwired: 1 in, 4 out]
              }
              frame True {
              }
            }
          }
          frame "Close" {
            n64 = property class="VI"(reference=w151, error in=w153) -> (reference out=w150:refnum<vi>, error out=w152:errorcluster, "Front Panel.Open"=w149:bool)
            n65 = case shown="True" w149 {
              tunnel: [w155 w158] -> w154
              tunnel: w152 -> [w155 w157]
              tunnel: w150 -> [_ w156]
              frame False {
              }
              frame True {
                n66 = invoke class="VI" method="FP.Close"(reference=w156, error in=w157) -> (error out=w158:errorcluster)  [unwired: 1 in, 2 out]
              }
            }
          }
        }
        n67 = call <vilib>:"Add State(s) to Queue__JKI_lib_State_Machine.vi"("State(s) in (\"\")"=w136) -> ("States Out"=w135:string)  [unwired: 14 in]
      }
      frame "---------- Macro ----------" {
        # "Do not put any code in this frame.\n(It is a separator no-op. You can make a copy of this frame to create a new Macro frame)"
        n68 = call <vilib>:"Add State(s) to Queue__JKI_lib_State_Machine.vi"("State(s) in (\"\")"=w162) -> ("States Out"=w161:string)  [unwired: 14 in]
      }
      frame "Macro: Initialize" {
        w164 = "Data: Initialize\nInitialize Core Data\nUI: Initialize\nUI: Front Panel State >> Open\n4461: SETUP"  # Data: Initialize Initialize Core Data UI: Initialize UI: Front Panel State >> Open 4461: SETUP
        # "Initialization Macro\n(This is called once, when the VI starts)"
        n69 = call <vilib>:"Add State(s) to Queue__JKI_lib_State_Machine.vi"("State(s) in Front (\"\")"=w164, "State(s) in (\"\")"=w167) -> ("States Out"=w166:string)  [unwired: 13 in]
      }
      frame "Macro: Exit" {
        w169 = FALSE ("EXIT")
        # "Exit Macro\n(This is called once, when the VI exits)"
        n70 = Unbundle By Name(w168) -> ("Core.Close Panel on Exit?"=w175:bool)
        n71 = local write "EXIT"(w169) -> ()
        n72 = local write "RESET"(w169) -> ()
        n73 = Select(t="UI: Front Panel State >> Close", s=w175, f="") -> (s? t:f=w172:string)
        n74 = call <vilib>:"Add State(s) to Queue__JKI_lib_State_Machine.vi"("State(s) in (\"\")"=w172, "State(s) at Back (\"\")"="Data: Cleanup\nExit") -> ("States Out"=w170:string)  [unwired: 13 in]
        n75 = call <vilib>:"Add State(s) to Queue__JKI_lib_State_Machine.vi"("State(s) in Front (\"\")"=w170, "State(s) in (\"\")"=w178) -> ("States Out"=w177:string)  [unwired: 13 in]
      }
      frame "---------- 4461----------" {
        n76 = call <vilib>:"Add State(s) to Queue__JKI_lib_State_Machine.vi"("State(s) in (\"\")"=w182) -> ("States Out"=w181:string)  [unwired: 14 in]
      }
      frame "4461: SETUP" {
        n77 = local read "Channels: AO"() -> (w206:T8)
        n78 = local read "Remote Mode"() -> (w191:bool)
        n79 = Unbundle By Name(w206) -> ("AO f (Hz)"=w184:dbl[])
        n80 = Unbundle By Name(w187) -> ("sampling info"=w188:cluster{"Fs":dbl, "#s":dbl})
        n81 = call "FGV - Remote.vi"("error in"=w193, "Function"=enum16{"write", "read"}."write", "Remote Mode"=w191) -> ("error out"=w192:errorcluster)  [unwired: 3 in, 1 out]
        n82 = Index Array(array=w184) -> (element=w183:dbl)  [unwired: 1 in]
        n83 = case shown="True" "auto block size" {
          tunnel: w188 -> [_ w213]
          tunnel: [w210 w214] -> w186
          tunnel: w183 -> [_ w212]
          frame False {
            n84 = local read "sampling info"() -> (w210:cluster{"Fs":i32, "#s":i32})
          }
          frame True {
            n85 = case shown="True" TRUE {
              tunnel: [w215 w228] -> w214
              tunnel: w213 -> [w215 w227]
              tunnel: w212 -> [_ w217]
              frame False {
                # "\"IV mode\""
              }
              frame True {
                n86 = Multiply(x="x", y=w217) -> (x*y=w226:dbl)
                n87 = In Range and Coerce(upper limit=204800.0, x=w226, lower limit=1000.0) -> (coerced(x)=w216:dbl)  [unwired: 1 out]
                n88 = call "Fs and Ns for integer periods.vi"("f_integer"=w217, "Fs"=w216) -> ("#s_integer"=w218:dbl, "Fs_integer"=w223:dbl)  [unwired: 8 in]
                n89 = In Range and Coerce(upper limit=204800.0, x=w223, lower limit=1000.0) -> (coerced(x)=w222:dbl)  [unwired: 1 out]
                n90 = Bundle By Name(cluster=w227, "Fs"=w222, "#s"=w218) -> (w228:cluster{"Fs":dbl, "#s":dbl})
                n91 = local write "sampling info"(w228) -> ()
              }
            }
          }
        }
        n92 = local read "Channels: Lockin"() -> (w196:T9)
        n93 = call "FGV - Configuration - lockin.vi"("error in"=w192, "Function"=enum16{"write", "read"}."write", "Channels: Lockin"=w196) -> ("error out"=w201:errorcluster)  [unwired: 3 in, 1 out]
        n94 = local read "Channels: AO"() -> (w195:T8)
        n95 = call "FGV - Configuration - Output.vi"("error in"=w201, "Function"=enum16{"write", "read"}."write", "Channels: AO"=w195) -> ("error out"=w200:errorcluster)  [unwired: 3 in, 1 out]
        n96 = call "FGV - Trigger.vi"("error in"=w200, "Function"=enum16{"write", "read"}."write", "Trigger"=TRUE) -> ("error out"=w189:errorcluster)  [unwired: 3 in, 1 out]
        n97 = local read "Gain"() -> (w194:dbl[])
        n98 = Bundle By Name(cluster=w187, "sampling info"=w186) -> (w185:T16)
        n99 = call <userlib>:"FGV - KH Gain.vi"("error in"=w189, "Function"=enum16{"write", "read"}."write", "Array"=w194) -> ("error out"=w197:errorcluster)  [unwired: 3 in, 1 out]
        n100 = call <vilib>:"Add State(s) to Queue__JKI_lib_State_Machine.vi"("State(s) in (\"\")"=w209, "State(s) at Back (\"\")"="4461: CREATE" ("State(s) at Back (\"\")")) -> ("States Out"=w208:string)  [unwired: 13 in]
      }
      frame "4461: CREATE" {
        n101 = local read "AO Configuration"() -> (w233:T6)
        n102 = local read "AI Configuration"() -> (w235:T7)
        n103 = local read "AI Buffer Size (S)"() -> (w241:i32)
        n104 = Unbundle By Name(w230) -> ("sampling info"=w231:cluster{"Fs":dbl, "#s":dbl})
        n105 = local read "Channels: AO"() -> (w242:T8)
        n106 = local read "simulate?"() -> (w229:bool)
        n107 = case shown="False" w229 {
          tunnel: w235 -> [w254 _]
          tunnel: w233 -> [w253 _]
          tunnel: [w252 w272] -> w240
          tunnel: w231 -> [w251 _]
          tunnel: [w250 w272] -> w239
          tunnel: w241 -> [w249 _]
          tunnel: [w248 dbl[] [] ("phase log")] -> w234
          tunnel: w242 -> [w247 _]
          tunnel: w236 -> [w246 w267]
          tunnel: [w245 w266] -> w232
          frame False {
            n108 = disable-structure shown="Default" {
              disable-tunnel: w254 -> [w264 _]
              disable-tunnel: w253 -> [w263 _]
              disable-tunnel: [w262 _] -> w252
              disable-tunnel: w251 -> [w259 _]
              disable-tunnel: [w261 _] -> w250
              disable-tunnel: w249 -> [w257 _]
              disable-tunnel: [w258 _] -> w248
              disable-tunnel: w247 -> [w260 _]
              disable-tunnel: w246 -> [w256 _]
              disable-tunnel: [w255 _] -> w245
              frame condition #0 (active) {
                n109 = call "4461 - Create IO Channels Parallel.vi"("error in"=w256, "AI Buffer Size (S)"=w257, "sampling info"=w259, "AO"=w260, "AO Configuration"=w263, "AI Configuration"=w264) -> ("AO Task"=w261:refnum<k21>[], "AI task"=w262:refnum<k21>[], "error out"=w255:errorcluster, "phase log"=w258:dbl[])  [unwired: 2 in]
              }
              frame condition #1 {
              }
            }
          }
          frame True {
            w272 = refnum<k21>[] [] ("AI task")
            # "simulate mode"
            n110 = Initialize Array(1.0 ("element"), 8 ("dimension size")) -> (w265:dbl[])
            n111 = call <userlib>:"FGV - KH Gain.vi"("error in"=w267, "Function"=enum16{"write", "read"}."write", "Array"=w265) -> ("error out"=w266:errorcluster)  [unwired: 3 in, 1 out]
            n112 = local write "Gain"(w265) -> ()
          }
        }
        n113 = local write "phase log"(w234) -> ()
        n114 = Bundle By Name(cluster=w230, "AI task"=w240, "AO task"=w239) -> (w238:T16)
        n115 = call <vilib>:"Add State(s) to Queue__JKI_lib_State_Machine.vi"("State(s) in (\"\")"=w244, "State(s) at Back (\"\")"="4461: FGV" ("State(s) at Back (\"\")")) -> ("States Out"=w243:string)  [unwired: 13 in]
      }
      frame "4461: FGV" {
        n116 = call "FGV - Remote.vi"("error in"=w295, "Function"=enum16{"write", "read"}."read") -> ("error out"=w294:errorcluster, "Remote Mode"=w275:bool)  [unwired: 4 in]
        n117 = local write "Remote Mode"(w275) -> ()
        n118 = call "FGV - Configuration - Output.vi"("error in"=w294, "Function"=enum16{"write", "read"}."read") -> ("error out"=w297:errorcluster, "Channels: AO 2"=w281:T8)  [unwired: 4 in]
        n119 = local read "Channels: AO"() -> (w285:T8)
        n120 = local read "Channels: Lockin"() -> (w293:T9)
        n121 = call "FGV - Configuration - lockin.vi"("error in"=w297, "Function"=enum16{"write", "read"}."read") -> ("error out"=w273:errorcluster, "Channels: Lockin 2"=w292:T9)  [unwired: 4 in]
        n122 = Not Equal?(x=w285, y=w281) -> (x != y?=w282:T19)
        n123 = Not Equal?(x=w293, y=w292) -> (x != y?=w291:T20)
        n124 = Unbundle(w282) -> ("AO amp (V)"=w283:bool[], "AO DC (V)"=w277:bool[], "AO f (Hz)"=w278:bool[], "AO phi (deg)"=w279:bool[], "function"=w280:bool[])
        n125 = Unbundle(w291) -> ("REF f (Hz)"=w290:bool[], "REF phi (deg)"=w289:bool[])
        n126 = for {
          tunnel: w283 -> [w312] mode=indexing
          tunnel: w277 -> [w311] mode=indexing
          tunnel: [w307] -> w284 mode=indexing
          tunnel: w280 -> [w310] mode=indexing
          tunnel: w279 -> [w309] mode=indexing
          tunnel: w278 -> [w308] mode=indexing
          n127 = Compound Arithmetic op=OR(w312, w311, w308, w309, w310) -> (w307:bool)
        }
        n128 = for {
          tunnel: w290 -> [w321] mode=indexing
          tunnel: w289 -> [w320] mode=indexing
          tunnel: [w319] -> w288 mode=indexing
          n129 = Compound Arithmetic op=OR(w321, w320) -> (w319:bool)
        }
        n130 = Or Array Elements(Boolean array=w284) -> (logical OR=w276:bool)
        n131 = Or Array Elements(Boolean array=w288) -> (logical OR=w287:bool)
        n132 = And(x=w276, y=w275) -> (x .and. y?=w274:bool)
        n133 = And(x=w287, y=w275) -> (x .and. y?=w286:bool)
        n134 = case shown="False" w274 {
          tunnel: w281 -> [_ w315]
          frame False {
            n135 = local read "Channels: AO"() -> (w313:T8)
            n136 = call "FGV - Configuration - Output.vi"("Function"=enum16{"write", "read"}."write", "Channels: AO"=w313) -> ()  [unwired: 4 in, 2 out]
          }
          frame True {
            n137 = property on="Channels: AO" class="Clust (strict)"("Val(Sgnl)"=w315) -> ()  [unwired: 2 in, 2 out]
          }
        }
        n138 = case shown="False" w286 {
          tunnel: w292 -> [_ w318]
          frame False {
            n139 = local read "Channels: Lockin"() -> (w316:T9)
            n140 = call "FGV - Configuration - lockin.vi"("Function"=enum16{"write", "read"}."write", "Channels: Lockin"=w316) -> ()  [unwired: 4 in, 2 out]
          }
          frame True {
            n141 = property on="Channels: Lockin" class="Clust (strict)"("Val(Sgnl)"=w318) -> ()  [unwired: 2 in, 2 out]
          }
        }
        n142 = call <userlib>:"FGV - KH Gain.vi"("error in"=w273, "Function"=enum16{"write", "read"}."read") -> ("error out"=w299:errorcluster, "Array 2"=w298:dbl[])  [unwired: 4 in]
        n143 = local write "Gain"(w298) -> ()
        n144 = call <vilib>:"Add State(s) to Queue__JKI_lib_State_Machine.vi"("State(s) in (\"\")"=w304, "State(s) at Back (\"\")"="4461: DATA" ("State(s) at Back (\"\")")) -> ("States Out"=w305:string)  [unwired: 13 in]
      }
      frame "4461: DATA" {
        w322 = waveform(dbl)[] [] ("Array out")
        n145 = Unbundle By Name(w331) -> ("sampling info"=w328:cluster{"Fs":dbl, "#s":dbl}, "AI task"=w330:refnum<k21>[])
        n146 = call-poly <userlib>:"Empty Array__ogtk.vi"("Array"=w330) -> ("Empty Array?"=w329:bool)  [unwired: 8 in]
        n147 = for {
          N: "Numeric" -> [_]
          tunnel: w343 -> [w372]
          tunnel: [w371] -> w342 mode=indexing
          tunnel: [w365] -> w334 mode=indexing
          tunnel: w331 -> [w362]
          tunnel: w328 -> [w361]
          tunnel: w329 -> [w359]
          shift-right: [w353] -> w332
          shift-left: w322 -> [w349]
          shift-right: [w352] -> w323
          shift-left: w322 -> [w350]
          shift-right: [w356] -> w324
          shift-left: w322 -> [w355]
          i -> [w348]
          n148 = First Call?() -> (First Call?: T/F=w373:bool)
          n149 = local read "measure offset"() -> (w370:bool)
          n150 = local read "Channels: AO"() -> (w366:T8)
          n151 = local read "Channels: Lockin"() -> (w367:T9)
          n152 = local read "reset signal"() -> (w374:bool)
          n153 = Or(x=w373, y=w374) -> (x .or. y?=w375:bool)
          n154 = Select(t=T8 {"AO amp (V)"=[0.0, 0.0, 0.0, 0.0, 0.0, 0.0, 0.0, 0.0], "AO DC (V)"=[0.0, 0.0, 0.0, 0.0, 0.0, 0.0, 0.04500000000000003, 0.0], "AO f (Hz)"=[0.4, 0.4, 0.4, 0.4, 0.4, 0.4, 0.4, 0.4], "AO phi (deg)"=[0.0, 0.0, 0.0, 0.0, 0.0, 0.0, 0.0, 0.0], "function"=[enum."Triangle Wave", enum."Sine Wave", enum."Sine Wave", enum."Sine Wave", enum."Sine Wave", enum."Sine Wave", enum."Sine Wave", enum."Sine Wave"]} ("Channels: AO"), s=w370, f=w366) -> (s? t:f=w369:T8)
          n155 = call "4461 - Create AO waveforms.vi"("error in (no error)"=w372, "sampling info"=w361, "reset signal"=w375, "AO"=w369) -> ("error out"=w364:errorcluster, "phase out"=w357:dbl[], "AO Array"=w363:waveform(dbl)[])  [unwired: 4 in, 1 out]
          n156 = call "4461 - Create Reference Waveforms.vi"("error in (no error)"=w372, "sampling info"=w361, "reset signal"=w375, "Lockin"=w367) -> ("error out"=w365:errorcluster, "AO Array"=w354:waveform(dbl)[])  [unwired: 4 in, 2 out]
          n157 = local read "simulate?"() -> (w360:bool)
          n158 = local write "phase log"(w357) -> ()
          n159 = Or(x=w359, y=w360) -> (x .or. y?=w358:bool)
          n160 = case shown="True" w358 {
            tunnel: [w396 w408] -> w347
            tunnel: w363 -> [w390 w406]
            tunnel: w361 -> [w391 w405]
            tunnel: w362 -> [w393 _]
            tunnel: w364 -> [w392 w407]
            tunnel: [w394 w407] -> w371
            tunnel: [w389 w406] -> w351
            frame False {
              n161 = Unbundle By Name(w393) -> ("AI task"=w395:refnum<k21>[], "AO task"=w388:refnum<k21>[])
              n162 = disable-structure shown="Default" {
                disable-tunnel: [w397 _] -> w396
                disable-tunnel: w390 -> [w398 w404]
                disable-tunnel: w391 -> [w399 _]
                disable-tunnel: w395 -> [w401 _]
                disable-tunnel: w392 -> [w403 _]
                disable-tunnel: [w402 _] -> w394
                disable-tunnel: [w398 w404] -> w389
                disable-tunnel: w388 -> [w400 _]
                frame condition #0 (active) {
                  n163 = call "4461 - AI AND AI - Read AND Write.vi"("AO Array"=w398, "error in (no error)"=w403, "sampling info"=w399, "AO Task"=w400, "AI task"=w401) -> ("error out"=w402:errorcluster, "Input Signals"=w397:waveform(dbl)[])  [unwired: 5 in]
                }
                frame condition #1 {
                }
              }
            }
            frame True {
              n164 = call "4461 Sim - Noise.vi"("data"=w406, "sampling info"=w405) -> ("Data"=w408:waveform(dbl)[])  [unwired: 5 in]
            }
          }
          "Signals Graph 2" <- w347
          n165 = case shown="1, Default" w348 {
            tunnel: w347 -> [w378 w387]
            tunnel: [w378 w386] -> w356
            tunnel: w355 -> [_ w385]
            tunnel: w354 -> [w376 w384]
            tunnel: [w376 w383] -> w353
            tunnel: [w377 w382] -> w352
            tunnel: w351 -> [w377 w381]
            tunnel: w350 -> [_ w380]
            tunnel: w349 -> [_ w379]
            frame 0 {
            }
            frame 1, Default {
              n166 = call "AppendWaveformArray.vi"("Array B"=w387, "Array A"=w385) -> ("Array out"=w386:waveform(dbl)[])  [unwired: 9 in]
              n167 = call "AppendWaveformArray.vi"("Array B"=w381, "Array A"=w380) -> ("Array out"=w382:waveform(dbl)[])  [unwired: 9 in]
              n168 = call "AppendWaveformArray.vi"("Array B"=w384, "Array A"=w379) -> ("Array out"=w383:waveform(dbl)[])  [unwired: 9 in]
            }
          }
        }
        n169 = Unbundle By Name(w328) -> ("Fs"=w327:dbl, "#s"=w326:dbl)
        n170 = Divide(x=w327, y=w326) -> ()  [unwired: 1 out]
        n171 = Index Array(array=w324) -> (element=w340:waveform(dbl))  [unwired: 1 in]
        n172 = Bundle By Name(cluster=w331, "Input Signals"=w324, "Ouput Signals"=w323, "REF"=w332) -> (w344:T16)
        n173 = Unbundle By Name(w340) -> ("Y"=w339:dbl[])
        n174 = local write "time since trigger"(0.0 ("time since trigger")) -> ()
        n175 = call-poly <userlib>:"Empty Array__ogtk.vi"("Array"=w339) -> ("Empty Array?"=w337:bool)  [unwired: 8 in]
        n176 = Merge Errors(w342, w334) -> (w341:errorcluster)
        n177 = Select(t="4461: RESET" ("State(s) at Back (\"\")"), s=w337, f="4461: MOD" ("State(s) at Back (\"\")")) -> (s? t:f=w336:string)
        n178 = call <vilib>:"Add State(s) to Queue__JKI_lib_State_Machine.vi"("State(s) in (\"\")"=w346, "State(s) at Back (\"\")"=w336) -> ("States Out"=w345:string)  [unwired: 13 in]
      }
      frame "4461: MOD" {
        w409 = TRUE ("averaging")
        n179 = Unbundle By Name(w411) -> ("Ouput Signals"=w423:waveform(dbl)[], "Input Signals"=w433:waveform(dbl)[], "REF"=w422:waveform(dbl)[])
        n180 = local read "decimating factor"() -> (w414:i32)
        n181 = call "decimate_waveforms.vi"("decimating factor"=w414, "averaging"=w409, "error in (no error)"=w428, "Input Signal"=w423) -> ("error out"=w427:errorcluster, "Decimated Waveforms"=w413:waveform(dbl)[])  [unwired: 6 in]
        n182 = call "decimate_waveforms.vi"("decimating factor"=w414, "averaging"=w409, "error in (no error)"=w428, "Input Signal"=w433) -> ("error out"=w430:errorcluster, "Decimated Waveforms"=w420:waveform(dbl)[])  [unwired: 6 in]
        n183 = call "decimate_waveforms.vi"("decimating factor"=w414, "averaging"=w409, "error in (no error)"=w428, "Input Signal"=w422) -> ("error out"=w429:errorcluster, "Decimated Waveforms"=w412:waveform(dbl)[])  [unwired: 6 in]
        n184 = local read "offsets"() -> (w434:dbl[])
        n185 = Subtract(x=w420, y=w434) -> (x-y=w419:waveform(dbl)[])
        n186 = Merge Errors(w427, w430, w429) -> (w425:errorcluster)
        n187 = case shown="False" "60 Hz prefilter" {
          tunnel: w419 -> [w442 w444]
          tunnel: [w442 w443] -> w418
          frame False {
          }
          frame True {
            n188 = call "Prefilter_60Hz_Notch.vi"("Array"=w444) -> ("Array 2"=w443:waveform(dbl)[])  [unwired: 10 in]
          }
        }
        n189 = local read "measure offset"() -> (w426:bool)
        n190 = local read "zero offset"() -> (w424:bool)
        n191 = Index Array(array=w412) -> (element=w432:waveform(dbl))  [unwired: 1 in]
        n192 = case shown="False" "LP prefilter" {
          tunnel: w418 -> [w438 w441]
          tunnel: [w438 w440] -> w417
          tunnel: "LP cutoff (Hz)" -> [_ w439]
          frame False {
          }
          frame True {
            n193 = call "Prefilter_LP.vi"("high cutoff freq [Hz]"=w439, "Array"=w441) -> ("Array 2"=w440:waveform(dbl)[])  [unwired: 9 in]
          }
        }
        n194 = Unbundle By Name(w432) -> ("dt"=w431:dbl)
        n195 = local write "dt"(w431) -> ()
        n196 = case shown="False" w426 {
          tunnel: w411 -> [w448 w453]
          frame False {
            n197 = Unbundle By Name(w448) -> ("Input Signals"=w447:waveform(dbl)[])
            n198 = for {
              tunnel: w447 -> [w450] mode=indexing
              tunnel: [w449] -> w446 mode=indexing
              n199 = call-poly <vilib>:"Mean.vi"("X"=w450) -> ("mean"=w449:dbl)  [unwired: 1 out]
            }
            n200 = local write "mean"(w446) -> ()
          }
          frame True {
            n201 = Unbundle By Name(w453) -> ("Input Signals"=w452:waveform(dbl)[])
            n202 = for {
              tunnel: w452 -> [w455] mode=indexing
              tunnel: [w454] -> w451 mode=indexing
              n203 = call-poly <vilib>:"Mean.vi"("X"=w455) -> ("mean"=w454:dbl)  [unwired: 1 out]
            }
            n204 = local write "offsets"(w451) -> ()
            n205 = local write "mean"(w451) -> ()
          }
        }
        n206 = case shown="False" w424 {
          frame False {
          }
          frame True {
            n207 = local write "offsets"(dbl[] [0.0, 0.0, 0.0, 0.0, 0.0, 0.0, 0.0, 0.0] ("offsets")) -> ()
          }
        }
        n208 = Bundle By Name(cluster=w411, "Ouput Signals"=w413, "Input Signals"=w417, "REF"=w412) -> (w435:T16)
        n209 = call <vilib>:"Add State(s) to Queue__JKI_lib_State_Machine.vi"("State(s) in (\"\")"=w437, "State(s) at Back (\"\")"="4461: PHASE" ("State(s) at Back (\"\")")) -> ("States Out"=w436:string)  [unwired: 13 in]
      }
      frame "4461: PHASE" {
        n210 = local read "Results\n(X, Y, R, Theta, mean)"() -> (w468:dbl[][])
        n211 = local read "autophase?\n(experimental)"() -> (w467:bool)
        n212 = local read "phase log"() -> (w469:dbl[])
        n213 = local read "Channels: Lockin"() -> (w465:T9)
        n214 = local read "Channels: AO"() -> (w464:T8)
        n215 = call "lockin - Set all f same.vi"("all  frequencies same?"="all  f same?", "Lockin"=w465, "AO"=w464) -> ("Lockin 2"=w462:T9, "AO 2"=w461:T8)  [unwired: 7 in]
        n216 = call "lockin - Set REF phase equals zero.vi"("reset REF phi to zero"="reset REF phi to zero", "Lockin"=w462, "AO"=w461) -> ("Lockin 2"=w457:T9, "AO 2"=w463:T8)  [unwired: 7 in]
        n217 = case shown="False" w467 {
          tunnel: w469 -> [_ w478]
          tunnel: w468 -> [_ w477]
          tunnel: w457 -> [w473 w475]
          tunnel: [w473 w474] -> w458
          frame False {
          }
          frame True {
            # "do this for EACH lockin...\n- replace PID array with PID SV\n-  advance \"results\" by 8?\n- this should go BEFORE REF\nwaveform is generated"
            n218 = Index Array(array=w477, index (col)=3 ("index (row)")) -> (element=w480:dbl[])  [unwired: 1 in]
            n219 = call "Simple PID Array.vi"("D"="D", "I"="I", "P"="P", "process variable"=w480) -> ("output value"=w484:dbl[])  [unwired: 7 in]
            n220 = Subtract(x=w478, y=w484) -> (x-y=w476:dbl[])
            n221 = Bundle By Name(cluster=w475, "REF phi (deg)"=w476) -> (w474:T9)
          }
        }
        n222 = local write "Channels: AO"(w463) -> ()
        n223 = local write "Channels: Lockin"(w458) -> ()
        n224 = call <vilib>:"Add State(s) to Queue__JKI_lib_State_Machine.vi"("State(s) in (\"\")"=w472, "State(s) at Back (\"\")"="4461: LOCKIN" ("State(s) at Back (\"\")")) -> ("States Out"=w471:string)  [unwired: 13 in]
      }
      frame "4461: LOCKIN" {
        n225 = event shown="[0] Timeout" {
          selector: _ -> [_ _ _ _ _ _]
          dyn-events: _ -> [_ _ _ _ _ _]
          timeout: 0 -> [_ _ _ _ _ _]
          tunnel: w490 -> [w549 w550 w559 w563 w569 w577]
          tunnel: [w548 w551 w561 w565 w571 w576] -> w487
          tunnel: w491 -> [w546 w553 w560 w566 w572 w574]
          tunnel: [w547 w554 w562 w564 w568 w575] -> w488
          tunnel: w489 -> [w547 w555 w562 w564 w568 w575]
          tunnel: [w546 w553 w560 w566 w572 w574] -> w486
          event Timeout {
            n226 = event-data() -> ()  [unwired: 1 in, 1 out]
            n227 = Unbundle By Name(w546) -> ("Ouput Signals"=w507:waveform(dbl)[], "Input Signals"=w496:waveform(dbl)[], "REF"=w509:waveform(dbl)[], "sampling info"=w519:cluster{"Fs":dbl, "#s":dbl})
            n228 = local read "TC (s)"() -> (w545:dbl)
            n229 = local read "mean"() -> (w535:dbl[])
            n230 = local read "order"() -> (w544:i32)
            n231 = local read "Gain"() -> (w529:dbl[])
            n232 = Divide(x=w496, y=w529) -> (x/y=w497:waveform(dbl)[])
            n233 = call "Display n or dt.vi"("Display n?"="Display n?", "Input Waveforms"=w507) -> ("Output Waveforms"=w510:waveform(dbl)[])  [unwired: 9 in]
            n234 = call "Display n or dt.vi"("Display n?"="Display n?", "Input Waveforms"=w496) -> ("Output Waveforms"=w512:waveform(dbl)[])  [unwired: 9 in]
            n235 = Divide(x=w535, y=w529) -> (x/y=w534:dbl[])
            n236 = call "decimate_waveforms.vi"("decimating factor"="decimate graph", "averaging"=FALSE, "Input Signal"=w510) -> ("Decimated Waveforms"=→"Reference Graph":waveform(dbl)[])  [unwired: 7 in, 1 out]
            n237 = Index Array(array=w497) -> (element=w493:waveform(dbl))  [unwired: 1 in]
            n238 = call "decimate_waveforms.vi"("decimating factor"="decimate graph", "averaging"=FALSE, "Input Signal"=w512) -> ("Decimated Waveforms"=→"Signals Graph":waveform(dbl)[])  [unwired: 7 in, 1 out]
            n239 = Get Date/Time In Seconds() -> (seconds since 1Jan1904=w506:timestamp)
            n240 = Unbundle By Name(w493) -> ("t0"=w522:timestamp)
            n241 = local write "current time"(w506) -> ()
            n242 = local read "save time"() -> (w505:timestamp)
            n243 = call "4461 - Lockin Engine.vi"("order"=w544, "TC (s)"=w545, "sampling info"=w519, "Reference In"=w509, "Signal in"=w497) -> ("Results (X,Y,R,Theta)"=w537:dbl[][])  [unwired: 5 in, 1 out]
            n244 = Transpose 2D Array(2D array=w537) -> (transposed array=w527:dbl[][])
            n245 = Build Array (concatenate)(w527, w534) -> (w536:dbl[][])
            n246 = call "FGV - Signals - Input.vi"("Function"=enum16{"write", "read"}."write", "input signal"=w497) -> ()  [unwired: 4 in, 2 out]
            n247 = local read "Channel"() -> (w541:dbl)
            n248 = local read "Display"() -> (w543:enum16{"X and Y", "R and Theta"})
            n249 = Subtract(x=w506, y=w505) -> (x-y=w504:dbl)
            n250 = Transpose 2D Array(2D array=w536) -> (transposed array=w498:dbl[][])
            "Results\n(X, Y, R, Theta, mean)" <- w498
            n251 = call "FGV - Signals - Output.vi"("Function"=enum16{"write", "read"}."write", "input signal"=w507) -> ()  [unwired: 4 in, 2 out]
            n252 = Get Waveform Attribute(7:w493) -> (2:→"names":string[])  [unwired: 3 in, 3 out]
            n253 = local read "Tab Control 2"() -> (w531:T1)
            n254 = call "format display.vi"("Channel"=w541, "Display"=w543, "Results (X,Y,R,Theta)"=w537, "t0"=w522) -> ("X/R"=→"X or R":dbl, "Array 2"=→"XY Graph":cluster{dbl[], dbl[]}[], "Y/Theta Array"=→"Display Y (or Theta)":waveform(dbl)[], "X/R Array"=→"Display X (or R)":waveform(dbl)[], "Y/R"=→"Y or Theta":dbl)  [unwired: 3 in]
            n255 = Greater?(x=w504, y="save interval (s)") -> ()  [unwired: 1 out]
            n256 = call "FGV - Lockin Results.vi"("Function"=enum16{"write", "read"}."write", "Input Signals"=w498) -> ()  [unwired: 4 in, 2 out]
            n257 = local read "Wait on Trigger"() -> (w538:bool)
            n258 = Equal?(x=w531, y=T15."PS" ("Tab Control 2")) -> (x = y?=w533:bool)
            n259 = Equal?(x=w531, y=T15."FFT" ("Tab Control 2")) -> (x = y?=w514:bool)
            n260 = Or(x=w514, y=w533) -> (x .or. y?=w532:bool)
            n261 = Select(t="4461: TRIGGER" ("State(s) at Back (\"\")"), s=w538, f="4461: FGV" ("State(s) at Back (\"\")")) -> (s? t:f=w525:string)
            n262 = Select(t="4461: FFT" ("State(s) at Back (\"\")"), s=w532, f=w525) -> (s? t:f=w501:string)
            n263 = Select(t="4461: SAVE", s=FALSE, f=w501) -> (s? t:f=w500:string)
            n264 = call <vilib>:"Add State(s) to Queue__JKI_lib_State_Machine.vi"("State(s) in (\"\")"=w549, "State(s) at Back (\"\")"=w500) -> ("States Out"=w548:string)  [unwired: 13 in]
          }
          event "Remote Mode": Value Change {
            n265 = event-data() -> ()  [unwired: 1 in, 6 out]
            n266 = local read "Remote Mode"() -> (w557:bool)
            n267 = call "FGV - Remote.vi"("error in"=w555, "Function"=enum16{"write", "read"}."write", "Remote Mode"=w557) -> ("error out"=w554:errorcluster)  [unwired: 3 in, 1 out]
            n268 = call <vilib>:"Add State(s) to Queue__JKI_lib_State_Machine.vi"("State(s) in (\"\")"=w550, "State(s) at Back (\"\")"="4461: FGV" ("State(s) at Back (\"\")")) -> ("States Out"=w551:string)  [unwired: 13 in]
          }
          event "simulate?": Value Change {
            n269 = event-data() -> ()  [unwired: 1 in, 6 out]
            n270 = call <vilib>:"Add State(s) to Queue__JKI_lib_State_Machine.vi"("State(s) in (\"\")"=w559, "State(s) at Back (\"\")"="4461: RESET") -> ("States Out"=w561:string)  [unwired: 13 in]
          }
          event "Save Data": Value Change {
            n271 = event-data() -> ()  [unwired: 1 in, 6 out]
            n272 = call <vilib>:"Add State(s) to Queue__JKI_lib_State_Machine.vi"("State(s) in (\"\")"=w563, "State(s) at Back (\"\")"="4461: SAVE") -> ("States Out"=w565:string)  [unwired: 13 in]
          }
          event "RESET": Value Change {
            n273 = event-data() -> ()  [unwired: 1 in, 6 out]
            n274 = call <vilib>:"Add State(s) to Queue__JKI_lib_State_Machine.vi"("State(s) in (\"\")"=w569, "State(s) at Back (\"\")"="4461: RESET") -> ("States Out"=w571:string)  [unwired: 13 in]
          }
          event "EXIT": Value Change {
            (unwired) "4461: SETUP"
            (unwired) "4461: RESET"
            # "Add other events to reset lockin (4461: RESET --> 4461 SETUP)"
            # "Exit Button Value Change (pressed) Event\n(this executes Macro: Exit to terminate the VI)"
            n275 = event-data() -> ()  [unwired: 1 in, 1 out]
            n276 = call <vilib>:"Add State(s) to Queue__JKI_lib_State_Machine.vi"("State(s) in (\"\")"=w577, "State(s) at Back (\"\")"="4461: EXIT\nMacro: Exit") -> ("States Out"=w576:string)  [unwired: 13 in]
          }
        }
      }
      frame "4461: FFT" {
        n277 = Unbundle By Name(w599) -> ("Input Signals"=w578:waveform(dbl)[])
        n278 = local read "Gain"() -> (w597:dbl[])
        n279 = Divide(x=w578, y=w597) -> (x/y=w586:waveform(dbl)[])
        n280 = property on="PS dB" class="WFGraph (strict)"("Active Cursor"=u32 1) -> ("Cursor.Cursor X"=w591:dbl)  [unwired: 2 in, 2 out]
        n281 = property on="PS dB" class="WFGraph (strict)"("Active Cursor"=u32 0) -> ("Cursor.Cursor X"=w592:dbl)  [unwired: 2 in, 2 out]
        n282 = call-poly <vilib>:"FFT Power Spectrum and PSD.vi"("window parameter"="window parameter", "export mode"="export mode", "averaging parameters"="averaging parameters", "restart averaging (F)"="restart averaging (F)", "dB On (F)"=TRUE, "window"="window", "time signals"=w586) -> ("averages completed"=→"averages\ncompleted":dbl, "averaging done"=→"averaging done":bool, "Power Spectrum / PSD"=w594:cluster{"f0":dbl, "df":dbl, "magnitude":dbl[]}[])  [unwired: 1 in, 1 out]
        "PS dB" <- w594
        n283 = for {
          tunnel: w594 -> [w619] mode=indexing
          tunnel: [w614] -> w593 mode=indexing
          n284 = Unbundle By Name(w619) -> ("df"=w621:dbl, "magnitude"=w620:dbl[])  [unwired: 1 out]
          n285 = Bundle By Name("dt"=w621, "Y"=w620) -> (w618:waveform(dbl))  [unwired: 1 in]
          n286 = call-poly <vilib>:"Waveform to XY Pairs.vi"("waveform in"=w618) -> ("XY pairs"=w617:cluster{"x":timestamp, "y":dbl}[])  [unwired: 8 in, 2 out]
          n287 = for {
            tunnel: w617 -> [w625] mode=indexing
            tunnel: [w623] -> w615 mode=indexing
            tunnel: [w622] -> w616 mode=indexing
            n288 = Unbundle(w625) -> ("x"=w624:timestamp, "y"=w623:dbl)
            n289 = To Double Precision Float(number=w624) -> (double precision float=w622:dbl)
          }
          n290 = Bundle(w616, w615) -> (w614:cluster{dbl[], dbl[]})  [unwired: 1 in]
        }
        n291 = Build Array(w592, w591) -> (w590:dbl[])
        n292 = for {
          tunnel: w593 -> [w613] mode=indexing
          tunnel: w590 -> [w612]
          tunnel: [w604] -> w589 mode=indexing
          n293 = Array Max & Min(array=w612) -> (max value=w611:dbl, min value=w609:dbl)  [unwired: 2 out]
          n294 = Unbundle(w613) -> (w610:dbl[], w608:dbl[])
          n295 = Threshold 1D Array(2:w611, 3:w610) -> (0:w607:dbl)  [unwired: 1 in]
          n296 = Threshold 1D Array(2:w609, 3:w610) -> (0:w606:dbl)  [unwired: 1 in]
          n297 = Subtract(x=w607, y=w606) -> (x-y=w605:dbl)
          n298 = Array Subset(array=w608, index=w606, length=w605) -> (w603:dbl[])
          n299 = Add Array Elements(numeric array=w603) -> (sum=w604:dbl)
        }
        n300 = Build Array(w589) -> (→"PS Chart":dbl[][])
        n301 = call <vilib>:"Add State(s) to Queue__JKI_lib_State_Machine.vi"("State(s) in (\"\")"=w602, "State(s) at Back (\"\")"="4461: FGV" ("State(s) at Back (\"\")")) -> ("States Out"=w600:string)  [unwired: 13 in]
      }
      frame "4461: TRIGGER" {
        # "Wait for Trigger signal from other VI"
        n302 = Get Date/Time In Seconds() -> (seconds since 1Jan1904=w632:timestamp)
        n303 = while {
          tunnel: w632 -> [w648]
          tunnel: [FALSE ("Trigger")] -> w631
          tunnel: w629 -> [w640]
          tunnel: [w639] -> w628
          stop <- w645 stop-if-true
          # "Initiate trigger (acquire data) if wating longer\nthan 10 seconds"
          n304 = Get Date/Time In Seconds() -> (seconds since 1Jan1904=w649:timestamp)
          n305 = Wait (ms)(milliseconds to wait=u32 100) -> ()  [unwired: 1 out]
          n306 = Subtract(x=w649, y=w648) -> (x-y=w636:dbl)
          n307 = Greater?(x=w636, y=10.0) -> (0:w646:bool)
          n308 = call "FGV - Trigger.vi"("error in"=w640, "Function"=enum16{"write", "read"}."read") -> ("error out"=w639:errorcluster, "Trigger 2"=w642:bool)  [unwired: 4 in]
          n309 = local write "time since trigger"(w636) -> ()
          n310 = local read "Wait on Trigger"() -> (w637:bool)
          n311 = Not(x=w637) -> (.not. x?=w638:bool)
          n312 = Compound Arithmetic op=OR(w638, w646, w642) -> (w645:bool)
        }
        n313 = call "FGV - Trigger.vi"("error in"=w628, "Function"=enum16{"write", "read"}."write", "Trigger"=w631) -> ("error out"=w627:errorcluster)  [unwired: 3 in, 1 out]
        n314 = call <vilib>:"Add State(s) to Queue__JKI_lib_State_Machine.vi"("State(s) in (\"\")"=w635, "State(s) at Back (\"\")"="4461: FGV" ("State(s) at Back (\"\")")) -> ("States Out"=w634:string)  [unwired: 13 in]
      }
      frame "4461: SAVE" {
        w651 = "FFT" ("filename")
        w650 = "signal" ("filename")
        # "Wait for Trigger signal from other VI"
        n315 = local read "PS dB"() -> (w669:cluster{"f0":dbl, "df":dbl, "magnitude":dbl[]}[])
        n316 = Get Date/Time In Seconds() -> (seconds since 1Jan1904=w659:timestamp)
        n317 = for {
          tunnel: w669 -> [w689] mode=indexing
          tunnel: [w684] -> w664 mode=indexing
          n318 = Unbundle By Name(w689) -> ("df"=w691:dbl, "magnitude"=w690:dbl[])  [unwired: 1 out]
          n319 = Bundle By Name("dt"=w691, "Y"=w690) -> (w688:waveform(dbl))  [unwired: 1 in]
          n320 = call-poly <vilib>:"Waveform to XY Pairs.vi"("waveform in"=w688) -> ("XY pairs"=w687:cluster{"x":timestamp, "y":dbl}[])  [unwired: 8 in, 2 out]
          n321 = for {
            tunnel: w687 -> [w695] mode=indexing
            tunnel: [w693] -> w685 mode=indexing
            tunnel: [w692] -> w686 mode=indexing
            n322 = Unbundle(w695) -> ("x"=w694:timestamp, "y"=w693:dbl)
            n323 = To Double Precision Float(number=w694) -> (double precision float=w692:dbl)
          }
          n324 = Bundle(w686, w685) -> (w684:cluster{dbl[], dbl[]})  [unwired: 1 in]
        }
        n325 = local read "path"() -> (w656:path)
        n326 = local write "save time"(w659) -> ()
        n327 = call "FGV - Signals - Input.vi"("error in"=w661, "Function"=enum16{"write", "read"}."read") -> ("error out"=w662:errorcluster, "input signal"=w668:waveform(dbl)[])  [unwired: 4 in]
        n328 = for {
          tunnel: [w676] -> w667 mode=indexing
          tunnel: w668 -> [w675] mode=indexing
          n329 = call-poly <vilib>:"Waveform to XY Pairs.vi"("waveform in"=w675) -> ("XY pairs"=w679:cluster{"x":timestamp, "y":dbl}[])  [unwired: 8 in, 2 out]
          n330 = for {
            tunnel: w679 -> [w683] mode=indexing
            tunnel: [w681] -> w677 mode=indexing
            tunnel: [w680] -> w678 mode=indexing
            n331 = Unbundle(w683) -> ("x"=w682:timestamp, "y"=w681:dbl)
            n332 = To Double Precision Float(number=w682) -> (double precision float=w680:dbl)
          }
          n333 = Bundle(w678, w677) -> (w676:cluster{dbl[], dbl[]})  [unwired: 1 in]
        }
        n334 = Format Date/Time String(time format string (%c)="%Y-%m-%d", seconds (now)=w659) -> (date/time string=w657:string)  [unwired: 1 in]
        n335 = Build Path(base path=w656, name or relative path=w657) -> (appended path=w654:path)
        n336 = Build Path(base path=w654, name or relative path=w650) -> (appended path=w653:path)
        n337 = call <userlib>:"LV to ITX XY AutoPlot.vi"("filename"=w650, "path"=w653, "Notes"="Notes", "XY Array"=w667, "wavenames (.Vx, etc)"=string[] ["ch0", "ch1", "ch2", "ch3", "ch4", "ch5", "ch6", "ch7"]) -> ()  [unwired: 10 in, 1 out]
        n338 = Build Path(base path=w654, name or relative path=w651) -> (appended path=w652:path)
        n339 = local write "Save Data"(FALSE ("SAVE DATA")) -> ()
        n340 = call <userlib>:"LV to ITX XY AutoPlot.vi"("filename"=w651, "path"=w652, "Notes"="Notes", "XY Array"=w664, "wavenames (.Vx, etc)"=string[] ["FFT0", "FFT1", "FFT2", "FFT3", "FFT4", "FFT5", "FFT6", "FFT7"], "X,Y Log"=i32[] [1, 1]) -> ()  [unwired: 9 in, 1 out]
        n341 = call <vilib>:"Add State(s) to Queue__JKI_lib_State_Machine.vi"("State(s) in (\"\")"=w674, "State(s) at Back (\"\")"="4461: FGV" ("State(s) at Back (\"\")")) -> ("States Out"=w673:string)  [unwired: 13 in]
      }
      frame "4461: RESET" {
        n342 = Unbundle By Name(w707) -> ("AI task"=w699:refnum<k21>[], "AO task"=w706:refnum<k21>[])
        n343 = local read "simulate?"() -> (w697:bool)
        n344 = call-poly <userlib>:"Empty Array__ogtk.vi"("Array"=w699) -> ("Empty Array?"=w698:bool)  [unwired: 8 in]
        n345 = Or(x=w697, y=w698) -> (x .or. y?=w696:bool)
        n346 = case shown="False" w696 {
          tunnel: w706 -> [w711 _]
          tunnel: w702 -> [w710 w739]
          tunnel: [w709 w739] -> w701
          tunnel: w699 -> [w708 _]
          frame False {
            n347 = disable-structure shown="Default" {
              disable-tunnel: w711 -> [w713 _]
              disable-tunnel: w710 -> [w714 _]
              disable-tunnel: [w715 _] -> w709
              disable-tunnel: w708 -> [w712 _]
              frame condition #0 (active) {
                n348 = for {
                  tunnel: w713 -> [w738] mode=indexing
                  tunnel: [w736] -> w720 mode=indexing
                  tunnel: w714 -> [w735]
                  tunnel: [w734] -> w717
                  n349 = call <vilib>:"DAQmx Stop Task.vi"("task/channels in"=w738, "error in"=w735) -> ("task out"=w736:refnum<k21>, "error out"=w734:errorcluster)  [unwired: 12 in]
                  n350 = Wait (ms)(milliseconds to wait=u32 50) -> ()  [unwired: 1 out]
                }
                n351 = for {
                  tunnel: w712 -> [w733] mode=indexing
                  tunnel: [w731] -> w716 mode=indexing
                  tunnel: w717 -> [w730]
                  tunnel: [w729] -> w719
                  n352 = call <vilib>:"DAQmx Stop Task.vi"("task/channels in"=w733, "error in"=w730) -> ("task out"=w731:refnum<k21>, "error out"=w729:errorcluster)  [unwired: 12 in]
                  n353 = Wait (ms)(milliseconds to wait=u32 50) -> ()  [unwired: 1 out]
                }
                n354 = for {
                  tunnel: w720 -> [w728] mode=indexing
                  tunnel: w719 -> [w726]
                  tunnel: [w725] -> w718
                  n355 = call <vilib>:"DAQmx Clear Task.vi"("task in"=w728, "error in"=w726) -> ("error out"=w725:errorcluster)  [unwired: 13 in]
                  n356 = Wait (ms)(milliseconds to wait=u32 50) -> ()  [unwired: 1 out]
                }
                n357 = for {
                  tunnel: w716 -> [w724] mode=indexing
                  tunnel: w718 -> [w722]
                  tunnel: [w721] -> w715
                  n358 = call <vilib>:"DAQmx Clear Task.vi"("task in"=w724, "error in"=w722) -> ("error out"=w721:errorcluster)  [unwired: 13 in]
                  n359 = Wait (ms)(milliseconds to wait=u32 50) -> ()  [unwired: 1 out]
                }
              }
              frame condition #1 {
              }
            }
          }
          frame True {
          }
        }
        n360 = local write "RESET"(FALSE ("EXIT")) -> ()
        n361 = call <vilib>:"Add State(s) to Queue__JKI_lib_State_Machine.vi"("State(s) in Front (\"\")"="4461: SETUP", "State(s) in (\"\")"=w705) -> ("States Out"=w703:string)  [unwired: 13 in]
      }
      frame "4461: EXIT" {
        n362 = Unbundle By Name(w747) -> ("AO task"=w743:refnum<k21>[], "AI task"=w744:refnum<k21>[])
        n363 = local read "simulate?"() -> (w741:bool)
        n364 = call-poly <userlib>:"Empty Array__ogtk.vi"("Array"=w743) -> ("Empty Array?"=w742:bool)  [unwired: 8 in]
        n365 = Or(x=w741, y=w742) -> (x .or. y?=w740:bool)
        n366 = case shown="False" w740 {
          tunnel: w743 -> [w755 _]
          tunnel: w746 -> [w754 w783]
          tunnel: [w753 w783] -> w745
          tunnel: w744 -> [w752 _]
          frame False {
            n367 = disable-structure shown="Default" {
              disable-tunnel: w755 -> [w763 _]
              disable-tunnel: w754 -> [w762 _]
              disable-tunnel: [w759 _] -> w753
              disable-tunnel: w752 -> [w756 _]
              frame condition #0 (active) {
                n368 = for {
                  tunnel: w756 -> [w782] mode=indexing
                  tunnel: [w780] -> w764 mode=indexing
                  tunnel: w762 -> [w779]
                  tunnel: [w778] -> w758
                  n369 = call <vilib>:"DAQmx Stop Task.vi"("task/channels in"=w782, "error in"=w779) -> ("task out"=w780:refnum<k21>, "error out"=w778:errorcluster)  [unwired: 12 in]
                  n370 = Wait (ms)(milliseconds to wait=u32 50) -> ()  [unwired: 1 out]
                }
                n371 = for {
                  tunnel: w763 -> [w777] mode=indexing
                  tunnel: [w775] -> w757 mode=indexing
                  tunnel: w758 -> [w774]
                  tunnel: [w773] -> w761
                  n372 = call <vilib>:"DAQmx Stop Task.vi"("task/channels in"=w777, "error in"=w774) -> ("task out"=w775:refnum<k21>, "error out"=w773:errorcluster)  [unwired: 12 in]
                  n373 = Wait (ms)(milliseconds to wait=u32 50) -> ()  [unwired: 1 out]
                }
                n374 = for {
                  tunnel: w764 -> [w772] mode=indexing
                  tunnel: w761 -> [w770]
                  tunnel: [w769] -> w760
                  n375 = call <vilib>:"DAQmx Clear Task.vi"("task in"=w772, "error in"=w770) -> ("error out"=w769:errorcluster)  [unwired: 13 in]
                  n376 = Wait (ms)(milliseconds to wait=u32 50) -> ()  [unwired: 1 out]
                }
                n377 = for {
                  tunnel: w757 -> [w768] mode=indexing
                  tunnel: w760 -> [w766]
                  tunnel: [w765] -> w759
                  n378 = call <vilib>:"DAQmx Clear Task.vi"("task in"=w768, "error in"=w766) -> ("error out"=w765:errorcluster)  [unwired: 13 in]
                  n379 = Wait (ms)(milliseconds to wait=u32 50) -> ()  [unwired: 1 out]
                }
              }
              frame condition #1 {
              }
            }
          }
          frame True {
          }
        }
        n380 = Initialize Array(w750, 8 ("dimension size")) -> (w748:i32[])
        n381 = local write "phase log"(w748) -> ()
      }
    }
  }
